vi "NEW Gas Rack MAIN (RT).vi"() -> ()   [LabVIEW 2013]
uses:
  TypeDef/DataCluster.ctl
  TypeDef/Controller Names.ctl
  RT subVIs/Controls/TraceCluster.ctl
  TypeDef/Command Cluster.ctl
  TCP/PC/Event Mode.ctl
  CAN Communication/CAN Mode.ctl
  TCP/RT/RTsend PCrecv CMD.ctl
  RT subVIs/Controls/Stream RT FIFO Mode.ctl
  TypeDef/TCP Cluster.ctl
  TypeDef/Stability Cluster.ctl
  <vilib>/FPGAPlugInAG/sbRIO-9626/niLvFpga_Open_sbRIO-9626.vi
  <vilib>/rvi/interface/common/dynamic/niFpgaDynamicAddResources.vi
  <vilib>/rvi/interface/common/niFpgaWaitOnOcc.vi
  <vilib>/Utility/error.llb/Error Cluster From Error Code.vi
  <vilib>/rvi/errors/niLvFpgaAdjustHostInterfaceError.vi
  <vilib>/FPGAPlugInAG/Dynamic/niLvFpga_Reset_Dynamic.vi
  <vilib>/FPGAPlugInAG/Dynamic/niLvFpga_Run_Dynamic.vi
  <vilib>/rvi/interface/nirviOpenFPGA/nirviOpenFPGA.xnode
  FPGA Bitfiles/New Gas Rack.lvbitx
  FPGA/NEW Gas Rack Main (FPGA).vi
  <vilib>/rvi/interface/nirviReadWriteControl/nirviReadWriteControl.xnode
  <vilib>/rvi/interface/nirviMethod/nirviMethod.xnode
  <vilib>/NI_Real-Time Target Support.lvlib
  <vilib>/rvi/interface/Simulation/niFpgaSimulationCallBeginRW.vi
  <vilib>/ptbypt/NI_PtbyPt.lvlib
  <vilib>/FPGAPlugInAG/Dynamic/niLvFpga_ReadFifo_Dynamic.vi
  <vilib>/rvi/errors/niLvFpgaMergeErrorWithErrorCode.vi
  <vilib>/Analysis/NI_AALBase.lvlib
  <vilib>/Analysis/3filter.llb/Butterworth Filter (DBL).vi
  NiFpgaLv.dll
panel:
  out "element":dbl
  out "output array":dbl[](array[numeric])
  out "x-y":u32
  in  "Load Cmd":bool
  in  "CMD to Load":T1
  out "time 3":dbl
  out "time 2":dbl
  out "time":dbl
  out "Ave Data Cluster":T2 {"Efficiency (%)" format="%#_6f"; "Speed (RPM)" format="%#.1f"; "Fuel Temp (C)" format="%.1f"; "Controller Current (A)" format="%.2f"; "Controller Voltage (V)" format="%.2f"; "Flow (L/H)" format="%.1f"; "Pressure (kPA)" format="%.1f"; "Pump Current (Arms)" format="%.2f"; "Pump Voltage (V)" format="%#.2f"}
  in  "Tab Control Config":enum32{"PID/slew", "Cal/Hidden"}(tab)
  in  "SaveConfig":bool
  in  "ControlArray":T3(array[cluster])
  in  "Cal Coeffs":dbl[][](array[numeric])
  in  "TraceCluster":T4
  out "Speed":dbl
  in  "Max Window":dbl=1400.0 format="%.4f"
  in  "Min Window":dbl=300.0 format="%.4f"
  in  "ave pts":i32=10
  in  "EnumV":enum16{"Pump", "Controller"}(ring)
  in  "CAN CMD":u16
  out "PWM Period (ticks)":u32
  out "Speed Loop Time":dbl
  out "Actual Loop Time 2":u32
  in  "Count 2(uS)":u32=35
  out "Actual Loop Time":u32
  in  "Count 1(uS)":u32=100
  in  "Set Threshold":bool
  in  "Threshold":fxp<+/-,24,7> format="%#_20g"
  in  "Hysteresis":fxp<+,10,6>
  in  "CtCuttoff":fxp<+,24,5>=2.5416698455810547
  in  "Brushed Speed":bool
  in  "Stream Stop":bool
  in  "CommSegs":i32
  out "PrevCalDate":dbl
  in  "CmdCluster":T1
  out "PresSig":dbl
  out "VSig":dbl
  in  "VDirect":dbl
  in  "DirectV?":bool
  in  "DirectPres?":bool
  in  "PresDirect":dbl
  in  "constant update?":bool
  in  "Deadhead?":bool
  in  "PS Enable":bool
  out "Controller Name":T5
  out "Inst Data Cluster":T2 {"Efficiency (%)" format="%.2f"; "Speed (RPM)" format="%#.0f"; "Fuel Temp (C)" format="%.1f"; "Controller Current (A)" format="%.2f"; "Controller Voltage (V)" format="%.2f"; "Flow (L/H)" format="%.1f"; "Pressure (kPA)" format="%.1f"; "Pump Current (Arms)" format="%.2f"; "Pump Voltage (V)" format="%.2f"}
  out "Total (%)":dbl
  in  "GraphTab":enum32{"Page 1", "Page 2"}(tab)
  out "WFG1":dbl[][](graph)
  out "WFG2":dbl[][](graph)
  out "WFG3":dbl[][](graph)
  out "WFG6":dbl[][](graph)
  out "WFG5":dbl[][](graph)
  out "WFG4":dbl[][](graph)
  # "Minimum slew rate is\n600 * step size. This would\nlimit the per cycle change\nto a step size.\n\nChanges were close to expected\nbut changed the PID slews to\nexpected timing rather than\nfinding the time and results\nwere exact.\n\nWas wrong about how the slew\nworks. Slew of 5 still creates\nresults with a stepsize of 0.1.\nIt will just not change every\ncycle but will keep track\nuntil necessary build up."
  # "Should be 0.1"
  # "No longer needed once FPGA is cleaned up"
  # "CalDate is frozen to 3/8/17"
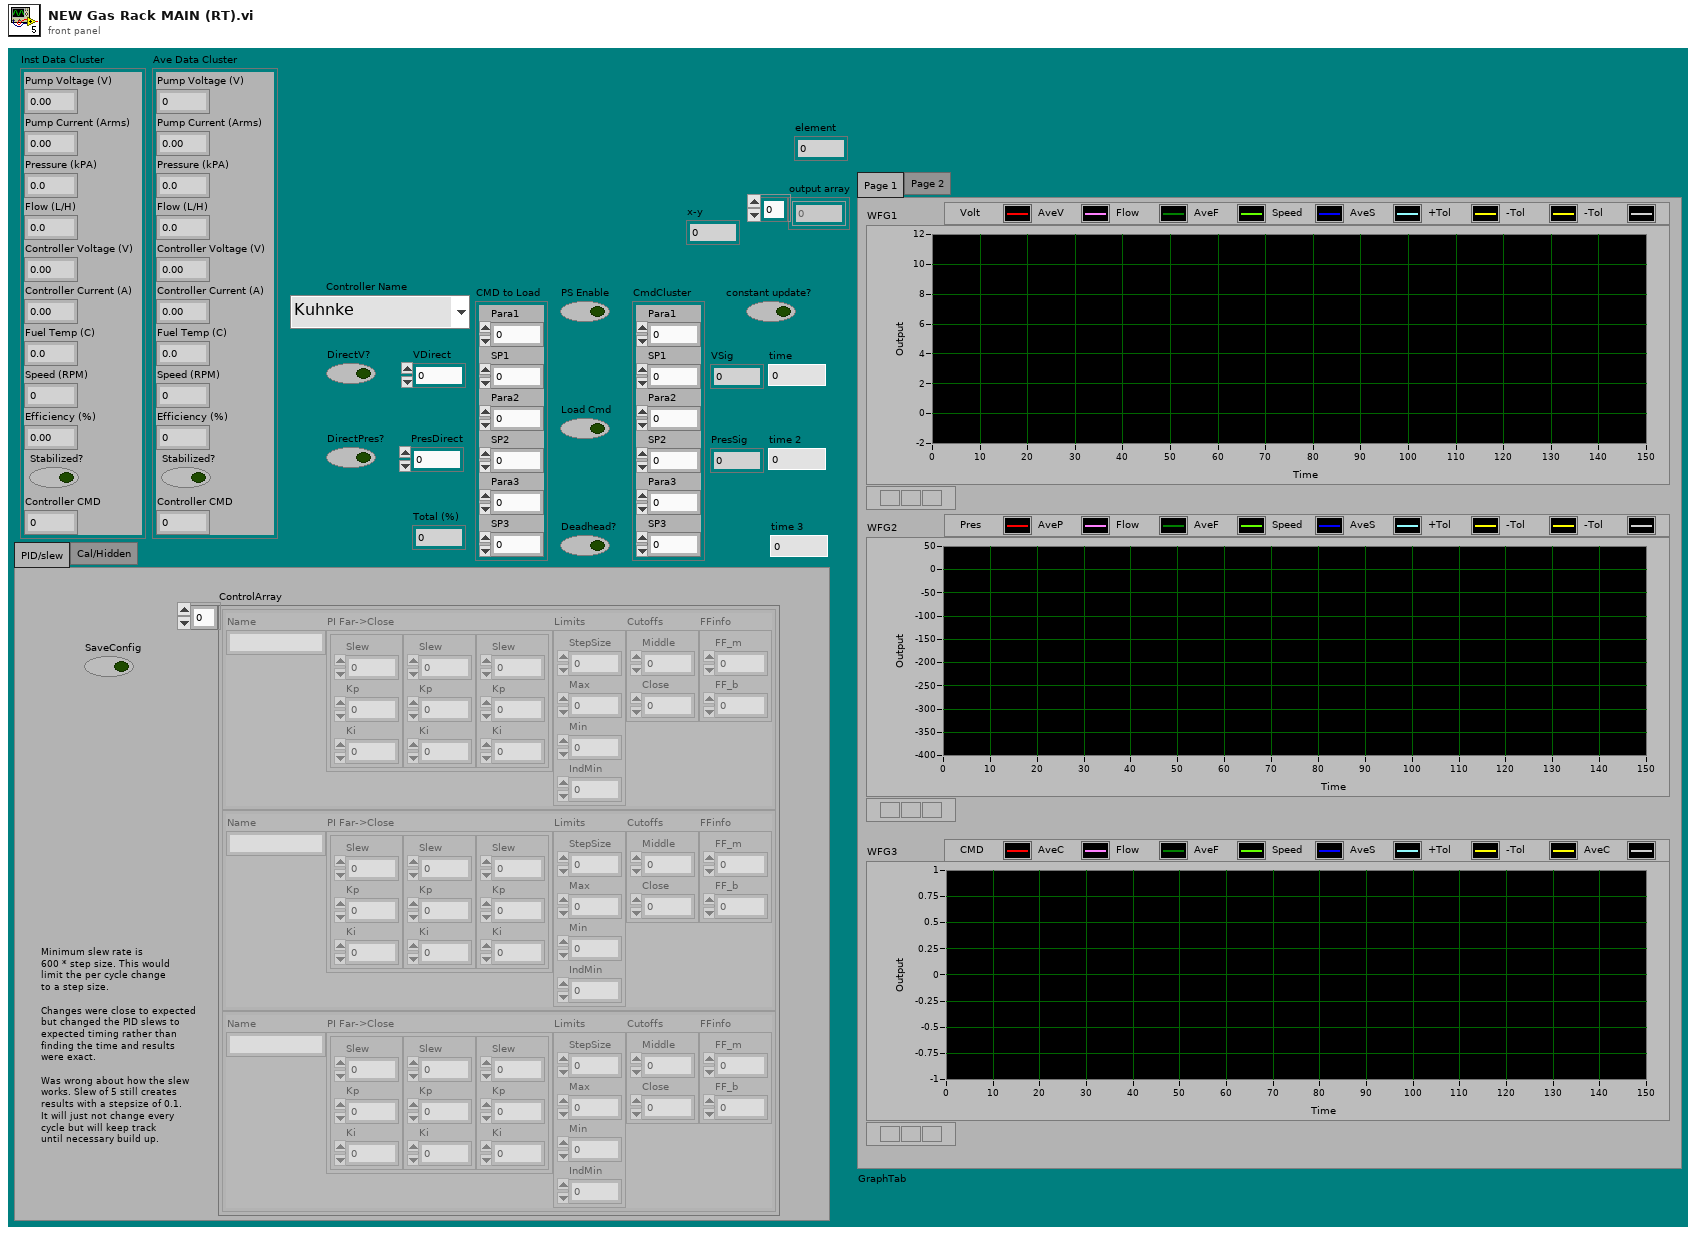
[diagram p1: front panel]
types:
  T1 = typedef "Command Cluster.ctl" = cluster{"Para1":i32, "SP1":dbl, "Para2":i32, "SP2":dbl, "Para3":i32, "SP3":dbl}
  T2 = typedef "DataCluster.ctl" = cluster{"Pump Voltage (V)":dbl, "Pump Current (Arms)":dbl, "Pressure (kPA)":dbl, "Flow (L/H)":dbl, "Controller Voltage (V)":dbl, "Controller Current (A)":dbl, "Fuel Temp (C)":dbl, "Speed (RPM)":dbl, "Efficiency (%)":dbl, "Stabilized?":bool, "Controller CMD":dbl}
  T3 = cluster{"Name":string, "PI Far->Close":cluster{"Slew":dbl, "Kp":dbl, "Ki":dbl}[], "Limits":cluster{"StepSize":dbl, "Max":dbl, "Min":dbl, "IndMin":dbl}, "Cutoffs":cluster{"Middle":dbl, "Close":dbl}, "FFinfo":cluster{"FF_m":dbl, "FF_b":dbl}}[]
  T4 = typedef "TraceCluster.ctl" = cluster{"PreTriggerPts":i32, "TotalPts":i32, "TriggerLvl":dbl, "PlotStyle":enum16{"Single - Rising Edge", "Single - Falling Edge", "Continuous", "Repeat - Rising Edge", "Repeat - Falling Edge"}, "TriggerChannel":i32, "TraceCtrl":bool}
  T5 = typedef "Controller Names.ctl" = enum16{"Kuhnke", "Helbako BLDC", "Conti", "Hella BLDC Screw", "Hella BLDC Turbine", "Helbako (old)", "TI PWM", "PSA", "Hella Gas", "Hella Diesel", "8 Comm", "10 Comm", "8 Comm Hella", "10 Comm Hella", "8 Comm Omron", "10 Comm Omron", "8 Comm Nissan", "10 Comm Nissan"}
  T6 = cluster{"Controller Name":T5, "CommSeg":i32, "PWM?":bool, "Frequency":i32, "Low Command":dbl, "High Command":dbl, "Stop Command":dbl, "Command Step":dbl, "Solenoid Stop?":bool, "Controller?":bool, "Name":string, "Indirect Nonzero CMD":dbl}[]
  T7 = cluster{"Controller Name":T5, "CommSeg":i32, "PWM?":bool, "Frequency":i32, "Low Command":dbl, "High Command":dbl, "Stop Command":dbl, "Command Step":dbl, "Solenoid Stop?":bool, "Controller?":bool, "Name":string, "Indirect Nonzero CMD":dbl}
  T8 = cluster{"Name":string, "PI Far->Close":cluster{"Slew":dbl, "Kp":dbl, "Ki":dbl}[], "Limits":cluster{"StepSize":dbl, "Max":dbl, "Min":dbl}, "Cutoffs":cluster{"Middle":dbl, "Close":dbl}, "FFinfo":cluster{"FF_m":dbl, "FF_b":dbl}}[]
  T9 = cluster{"Stability Reads":i32, "Stability1":i32, "Stability2":i32, "Stability3":i32}
  T10 = typedef "RTsend PCrecv CMD.ctl" = enum16{"Data", "Connected?", "CalFileDate"}
  T11 = typedef "CAN Mode.ctl" = enum16{"Init", "Read", "Write", "Close"}
  T12 = typedef "Event Mode.ctl" = enum16{"Init", "Get", "Set", "Destroy"}
  T13 = cluster{"CommandCluster":T1, "Deadhead?":bool, "PI Rate (sec)":dbl, "PI Timer":dbl, "FPGA Data Rate (sec)":dbl, "FPGA Data Timer":dbl, "PC Data Rate (sec)":dbl, "PC Data Timer":dbl, "InstDataCluster":T2, "Controller":cluster{"Controller Name":T5, "CommSeg":i32, "PWM?":bool, "Frequency":i32, "Low Command":dbl, "High Command":dbl, "Stop Command":dbl, "Command Step":dbl, "Solenoid Stop?":bool, "Controller?":bool, "Name":string, "Indirect Nonzero CMD":dbl}, "PWM Period (ticks)":u32, "Tolerances":dbl[], "Cal Coeffs":dbl[][], "EnumV":enum16{"Pump", "Controller"}, "PS Enable":bool, "StabilityCluster":cluster{"Stability Reads":i32, "Stability1":i32, "Stability2":i32, "Stability3":i32}, "AveDataCluster":T2, "CMD Scaler":dbl, "ControlArray":cluster{"Name":string, "PI Far->Close":cluster{"Slew":dbl, "Kp":dbl, "Ki":dbl}[], "Limits":cluster{"StepSize":dbl, "Max":dbl, "Min":dbl, "IndMin":dbl}, "Cutoffs":cluster{"Middle":dbl, "Close":dbl}, "FFinfo":cluster{"FF_m":dbl, "FF_b":dbl}}[], "Controller List":cluster{"Controller Name":T5, "CommSeg":i32, "PWM?":bool, "Frequency":i32, "Low Command":dbl, "High Command":dbl, "Stop Command":dbl, "Command Step":dbl, "Solenoid Stop?":bool, "Controller?":bool, "Name":string, "Indirect Nonzero CMD":dbl}[], "VandPLimit":dbl[]}
  T14 = typedef "TCP Cluster.ctl" = cluster{"Command":string, "FlattenedData":string}
  T15 = typedef "Stream RT FIFO Mode.ctl" = enum16{"Create", "Write", "Read", "Delete"}
  T16 = typedef "PCsend RTrecv CMD.ctl" = enum16{"ConnSettings", "Connect", "CMD", "Controller", "PSenable", "ReqCalDate", "Tolerances", "Stable Trigger", "Stop", "VPLimits"}
  T17 = typedef "Stability Cluster.ctl" = cluster{"Voltage Tolerances":dbl, "Pressure Tolerances":dbl, "Flow Tolerances":dbl, "Speed Tolerances":dbl, "Stable Count (sec)":dbl}
  T18 = cluster{"Pump Voltage":fxp<+/-,25,15>, "Pump Current":fxp<+/-,25,15>, "Pressure":fxp<+/-,25,15>, "Flow":fxp<+/-,25,15>, "Controller Voltage":fxp<+/-,25,15>, "Controller Current":fxp<+/-,25,15>, "Temperature":fxp<+/-,25,15>, "Speed":fxp<+/-,25,15>}
  T19 = cluster{"[0]":dbl, "[1]":dbl, "[2]":dbl, "[3]":dbl, "[4]":dbl, "[5]":dbl, "[6]":dbl, "[7]":dbl}
  T20 = typedef "NI_Real-Time Target Support.lvlib/RT CPU Load.ctl" = cluster{"Total (%)":dbl, "Time Critical (%)":dbl, "Timed Structures (%)":dbl, "High (%)":dbl, "Above Normal (%)":dbl, "Normal (%)":dbl, "Background (%)":dbl, "Idle (%)":dbl, "ISR (%)":dbl}
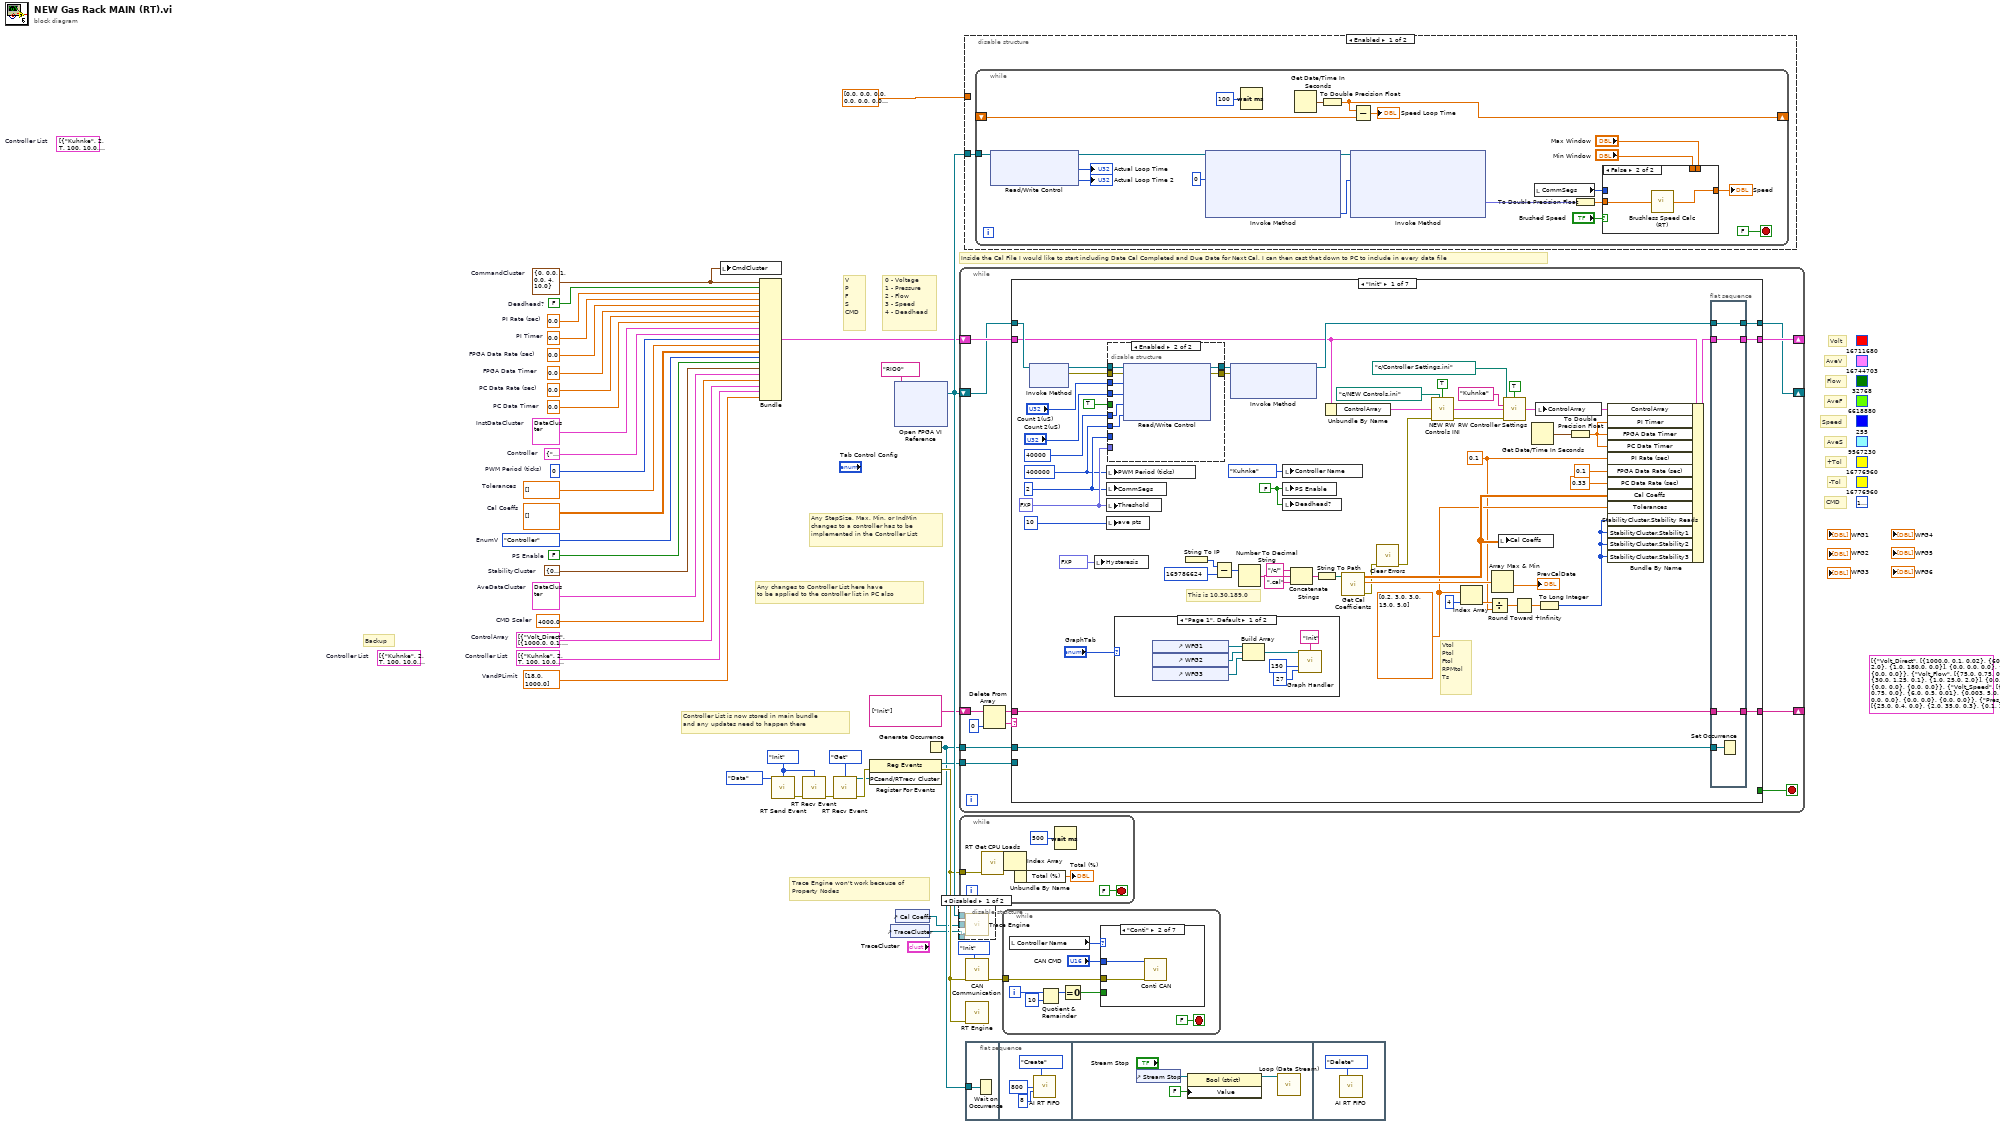
[diagram p0: block diagram]
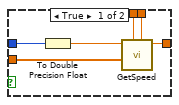
[diagram p2: hidden frame]
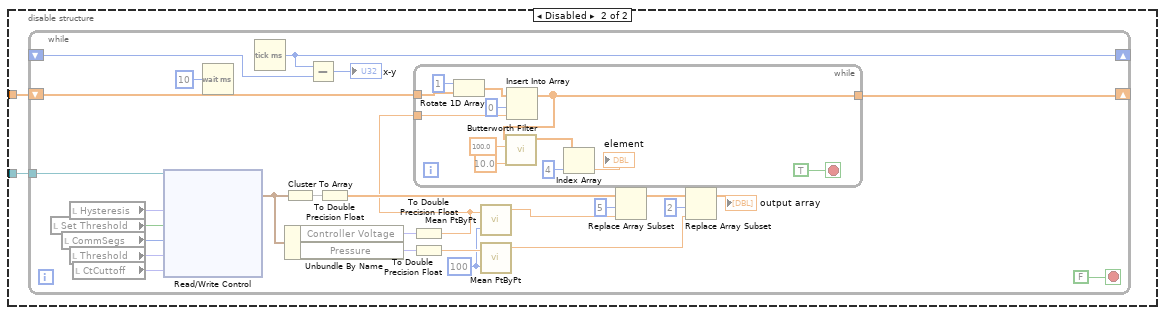
[diagram p3: hidden frame]
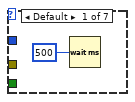
[diagram p5: hidden frame]
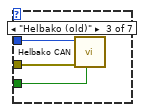
[diagram p6: hidden frame]
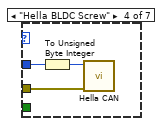
[diagram p7: hidden frame]
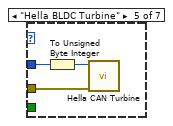
[diagram p8: hidden frame]
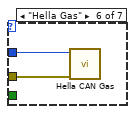
[diagram p9: hidden frame]
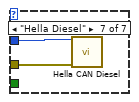
[diagram p10: hidden frame]
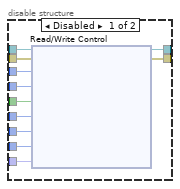
[diagram p11: hidden frame]
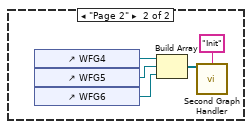
[diagram p12: hidden frame]
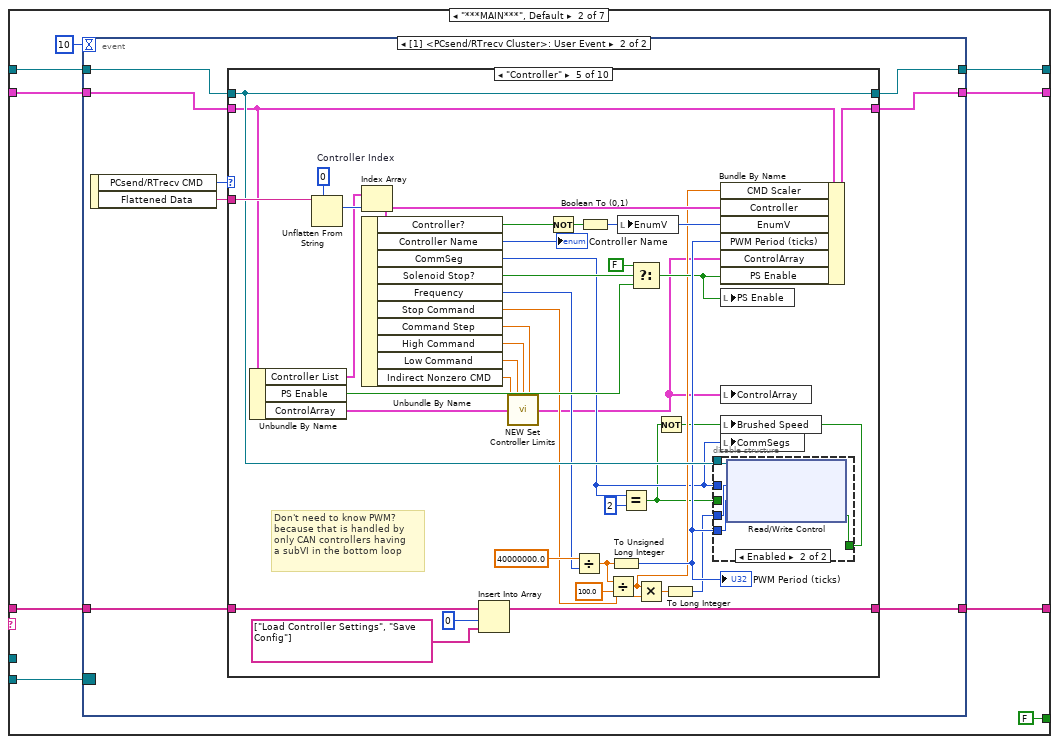
[diagram p13: hidden frame]
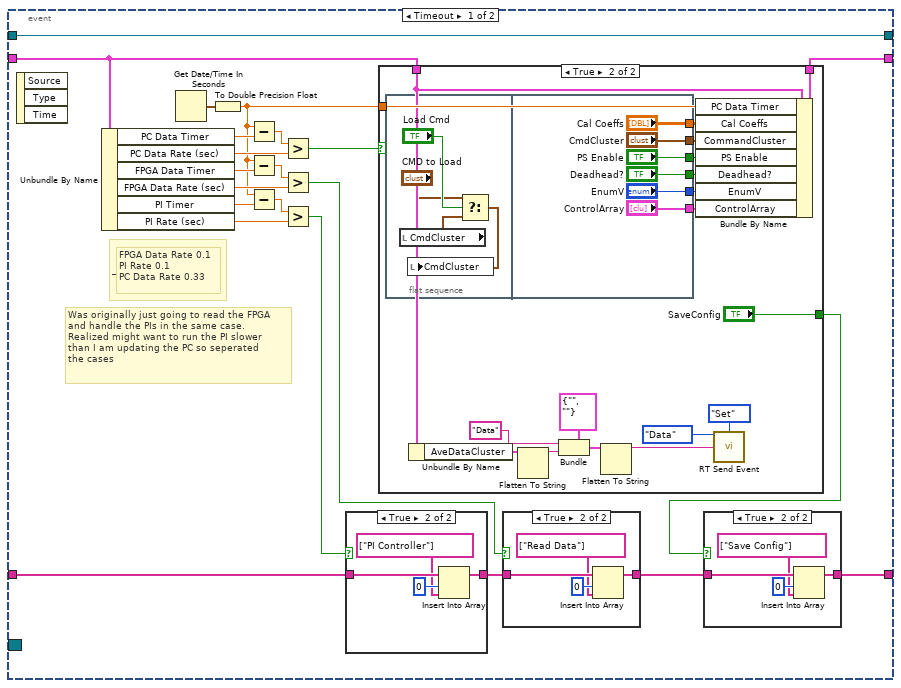
[diagram p14: hidden frame]
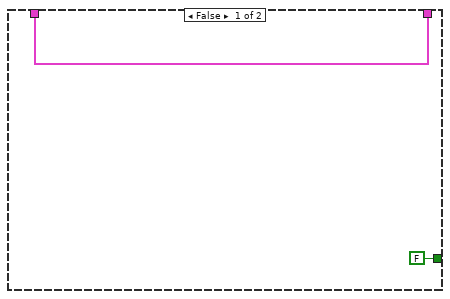
[diagram p18: hidden frame]
diagram:
  (unwired) T6 [{"Controller Name"=enum."Kuhnke", "CommSeg"=2, "PWM?"=TRUE, "Frequency"=100, "Low Command"=10.0, "High Command"=90.0, "Stop Command"=10.0, "Command Step"=0.1, "Solenoid Stop?"=FALSE, "Controller?"=TRUE, "Name"="Kuhnke", "Indirect Nonzero CMD"=15.0}, {"Controller Name"=enum."Helbako BLDC", "CommSeg"=2, "PWM?"=TRUE, "Frequency"=100, "Low Command"=10.0, "High Command"=90.0, "Stop Command"=10.0, "Command Step"=0.1, "Solenoid Stop?"=FALSE, "Controller?"=TRUE, "Name"="Helbako BLDC", "Indirect Nonzero CMD"=15.0}, {"Controller Name"=enum."Conti", "CommSeg"=2, "PWM?"=FALSE, "Frequency"=100, "Low Command"=0.0, "High Command"=800.0, "Stop Command"=0.0, "Command Step"=1.0, "Solenoid Stop?"=FALSE, "Controller?"=TRUE, "Name"="Conti", "Indirect Nonzero CMD"=0.0}, {"Controller Name"=enum."Hella BLDC Screw", "CommSeg"=2, "PWM?"=FALSE, "Frequency"=100, "Low Command"=0.0, "High Command"=100.0, "Stop Command"=0.0, "Command Step"=1.0, "Solenoid Stop?"=FALSE, "Controller?"=TRUE, "Name"="Hella BLDC Screw", "Indirect Nonzero CMD"=10.0}, {"Controller Name"=enum."Hella BLDC Turbine", "CommSeg"=2, "PWM?"=FALSE, "Frequency"=100, "Low Command"=0.0, "High Command"=100.0, "Stop Command"=0.0, "Command Step"=1.0, "Solenoid Stop?"=FALSE, "Controller?"=TRUE, "Name"="Hella BLDC Turbine", "Indirect Nonzero CMD"=10.0}, {"Controller Name"=enum."Helbako (old)", "CommSeg"=2, "PWM?"=FALSE, "Frequency"=100, "Low Command"=0.0, "High Command"=100.0, "Stop Command"=0.0, "Command Step"=0.1, "Solenoid Stop?"=FALSE, "Controller?"=TRUE, "Name"="Helbako (old)", "Indirect Nonzero CMD"=0.0}, {"Controller Name"=enum."TI PWM", "CommSeg"=2, "PWM?"=TRUE, "Frequency"=100, "Low Command"=0.0, "High Command"=100.0, "Stop Command"=0.0, "Command Step"=0.1, "Solenoid Stop?"=FALSE, "Controller?"=TRUE, "Name"="TI PWM", "Indirect Nonzero CMD"=0.0}, {"Controller Name"=enum."PSA", "CommSeg"=2, "PWM?"=TRUE, "Frequency"=100, "Low Command"=5.0, "High Command"=95.0, "Stop Command"=5.0, "Command Step"=0.1, "Solenoid Stop?"=FALSE, "Controller?"=TRUE, "Name"="PSA", "Indirect Nonzero CMD"=5.0}, {"Controller Name"=enum."Hella Gas", "CommSeg"=2, "PWM?"=FALSE, "Frequency"=100, "Low Command"=0.0, "High Command"=800.0, "Stop Command"=0.0, "Command Step"=1.0, "Solenoid Stop?"=TRUE, "Controller?"=TRUE, "Name"="Hella Gas", "Indirect Nonzero CMD"=0.0}, {"Controller Name"=enum."Hella Diesel", "CommSeg"=10, "PWM?"=FALSE, "Frequency"=100, "Low Command"=370.0, "High Command"=461.0, "Stop Command"=370.0, "Command Step"=1.0, "Solenoid Stop?"=TRUE, "Controller?"=TRUE, "Name"="Hella Diesel", "Indirect Nonzero CMD"=370.0}, {"Controller Name"=enum."8 Comm", "CommSeg"=8, "PWM?"=FALSE, "Frequency"=150, "Low Command"=0.0, "High Command"=1.0, "Stop Command"=0.0, "Command Step"=1.0, "Solenoid Stop?"=FALSE, "Controller?"=FALSE, "Name"="8 Comm", "Indirect Nonzero CMD"=0.0}, {"Controller Name"=enum."10 Comm", "CommSeg"=10, "PWM?"=FALSE, "Frequency"=150, "Low Command"=0.0, "High Command"=1.0, "Stop Command"=0.0, "Command Step"=1.0, "Solenoid Stop?"=FALSE, "Controller?"=FALSE, "Name"="10 Comm", "Indirect Nonzero CMD"=0.0}, {"Controller Name"=enum."8 Comm Hella", "CommSeg"=8, "PWM?"=TRUE, "Frequency"=150, "Low Command"=0.0, "High Command"=50.0, "Stop Command"=80.0, "Command Step"=0.1, "Solenoid Stop?"=FALSE, "Controller?"=TRUE, "Name"="8 Comm Hella", "Indirect Nonzero CMD"=0.0}, {"Controller Name"=enum."10 Comm Hella", "CommSeg"=10, "PWM?"=TRUE, "Frequency"=150, "Low Command"=0.0, "High Command"=50.0, "Stop Command"=80.0, "Command Step"=0.1, "Solenoid Stop?"=FALSE, "Controller?"=TRUE, "Name"="10 Comm Hella", "Indirect Nonzero CMD"=0.0}, {"Controller Name"=enum."8 Comm Omron", "CommSeg"=8, "PWM?"=TRUE, "Frequency"=150, "Low Command"=5.0, "High Command"=50.0, "Stop Command"=75.0, "Command Step"=0.1, "Solenoid Stop?"=FALSE, "Controller?"=TRUE, "Name"="8 Comm Omron", "Indirect Nonzero CMD"=5.0}, {"Controller Name"=enum."10 Comm Omron", "CommSeg"=10, "PWM?"=TRUE, "Frequency"=150, "Low Command"=5.0, "High Command"=50.0, "Stop Command"=75.0, "Command Step"=0.1, "Solenoid Stop?"=FALSE, "Controller?"=TRUE, "Name"="10 Comm Omron", "Indirect Nonzero CMD"=5.0}, {"Controller Name"=enum."8 Comm Nissan", "CommSeg"=8, "PWM?"=TRUE, "Frequency"=10, "Low Command"=50.0, "High Command"=90.0, "Stop Command"=50.0, "Command Step"=0.1, "Solenoid Stop?"=TRUE, "Controller?"=TRUE, "Name"="8 Comm Nissan", "Indirect Nonzero CMD"=50.0}, {"Controller Name"=enum."10 Comm Nissan", "CommSeg"=10, "PWM?"=TRUE, "Frequency"=10, "Low Command"=50.0, "High Command"=90.0, "Stop Command"=50.0, "Command Step"=0.1, "Solenoid Stop?"=TRUE, "Controller?"=TRUE, "Name"="10 Comm Nissan", "Indirect Nonzero CMD"=50.0}]  # Controller List
  w2 = T6 [{"Controller Name"=enum."Kuhnke", "CommSeg"=2, "PWM?"=TRUE, "Frequency"=100, "Low Command"=10.0, "High Command"=90.0, "Stop Command"=10.0, "Command Step"=0.1, "Solenoid Stop?"=FALSE, "Controller?"=TRUE, "Name"="Kuhnke", "Indirect Nonzero CMD"=15.0}, {"Controller Name"=enum."Helbako BLDC", "CommSeg"=2, "PWM?"=TRUE, "Frequency"=100, "Low Command"=10.0, "High Command"=90.0, "Stop Command"=10.0, "Command Step"=0.1, "Solenoid Stop?"=FALSE, "Controller?"=TRUE, "Name"="Helbako BLDC", "Indirect Nonzero CMD"=15.0}, {"Controller Name"=enum."Conti", "CommSeg"=2, "PWM?"=FALSE, "Frequency"=100, "Low Command"=0.0, "High Command"=800.0, "Stop Command"=0.0, "Command Step"=1.0, "Solenoid Stop?"=FALSE, "Controller?"=TRUE, "Name"="Conti", "Indirect Nonzero CMD"=0.0}, {"Controller Name"=enum."Hella BLDC Screw", "CommSeg"=2, "PWM?"=FALSE, "Frequency"=100, "Low Command"=0.0, "High Command"=100.0, "Stop Command"=0.0, "Command Step"=1.0, "Solenoid Stop?"=FALSE, "Controller?"=TRUE, "Name"="Hella BLDC Screw", "Indirect Nonzero CMD"=10.0}, {"Controller Name"=enum."Hella BLDC Turbine", "CommSeg"=2, "PWM?"=FALSE, "Frequency"=100, "Low Command"=0.0, "High Command"=100.0, "Stop Command"=0.0, "Command Step"=1.0, "Solenoid Stop?"=FALSE, "Controller?"=TRUE, "Name"="Hella BLDC Turbine", "Indirect Nonzero CMD"=10.0}, {"Controller Name"=enum."Helbako (old)", "CommSeg"=2, "PWM?"=FALSE, "Frequency"=100, "Low Command"=0.0, "High Command"=100.0, "Stop Command"=0.0, "Command Step"=0.1, "Solenoid Stop?"=FALSE, "Controller?"=TRUE, "Name"="Helbako (old)", "Indirect Nonzero CMD"=0.0}, {"Controller Name"=enum."TI PWM", "CommSeg"=2, "PWM?"=TRUE, "Frequency"=100, "Low Command"=0.0, "High Command"=100.0, "Stop Command"=0.0, "Command Step"=0.1, "Solenoid Stop?"=FALSE, "Controller?"=TRUE, "Name"="TI PWM", "Indirect Nonzero CMD"=0.0}, {"Controller Name"=enum."PSA", "CommSeg"=2, "PWM?"=TRUE, "Frequency"=100, "Low Command"=5.0, "High Command"=95.0, "Stop Command"=5.0, "Command Step"=0.1, "Solenoid Stop?"=FALSE, "Controller?"=TRUE, "Name"="PSA", "Indirect Nonzero CMD"=5.0}, {"Controller Name"=enum."Hella Gas", "CommSeg"=2, "PWM?"=FALSE, "Frequency"=100, "Low Command"=0.0, "High Command"=800.0, "Stop Command"=0.0, "Command Step"=1.0, "Solenoid Stop?"=TRUE, "Controller?"=TRUE, "Name"="Hella Gas", "Indirect Nonzero CMD"=0.0}, {"Controller Name"=enum."Hella Diesel", "CommSeg"=10, "PWM?"=FALSE, "Frequency"=100, "Low Command"=370.0, "High Command"=461.0, "Stop Command"=370.0, "Command Step"=1.0, "Solenoid Stop?"=TRUE, "Controller?"=TRUE, "Name"="Hella Diesel", "Indirect Nonzero CMD"=370.0}, {"Controller Name"=enum."8 Comm", "CommSeg"=8, "PWM?"=FALSE, "Frequency"=150, "Low Command"=0.0, "High Command"=1.0, "Stop Command"=0.0, "Command Step"=1.0, "Solenoid Stop?"=FALSE, "Controller?"=FALSE, "Name"="8 Comm", "Indirect Nonzero CMD"=0.0}, {"Controller Name"=enum."10 Comm", "CommSeg"=10, "PWM?"=FALSE, "Frequency"=150, "Low Command"=0.0, "High Command"=1.0, "Stop Command"=0.0, "Command Step"=1.0, "Solenoid Stop?"=FALSE, "Controller?"=FALSE, "Name"="10 Comm", "Indirect Nonzero CMD"=0.0}, {"Controller Name"=enum."8 Comm Hella", "CommSeg"=8, "PWM?"=TRUE, "Frequency"=150, "Low Command"=0.0, "High Command"=50.0, "Stop Command"=80.0, "Command Step"=0.1, "Solenoid Stop?"=FALSE, "Controller?"=TRUE, "Name"="8 Comm Hella", "Indirect Nonzero CMD"=0.0}, {"Controller Name"=enum."10 Comm Hella", "CommSeg"=10, "PWM?"=TRUE, "Frequency"=150, "Low Command"=0.0, "High Command"=50.0, "Stop Command"=80.0, "Command Step"=0.1, "Solenoid Stop?"=FALSE, "Controller?"=TRUE, "Name"="10 Comm Hella", "Indirect Nonzero CMD"=0.0}, {"Controller Name"=enum."8 Comm Omron", "CommSeg"=8, "PWM?"=TRUE, "Frequency"=150, "Low Command"=5.0, "High Command"=50.0, "Stop Command"=75.0, "Command Step"=0.1, "Solenoid Stop?"=FALSE, "Controller?"=TRUE, "Name"="8 Comm Omron", "Indirect Nonzero CMD"=5.0}, {"Controller Name"=enum."10 Comm Omron", "CommSeg"=10, "PWM?"=TRUE, "Frequency"=150, "Low Command"=5.0, "High Command"=50.0, "Stop Command"=75.0, "Command Step"=0.1, "Solenoid Stop?"=FALSE, "Controller?"=TRUE, "Name"="10 Comm Omron", "Indirect Nonzero CMD"=5.0}, {"Controller Name"=enum."8 Comm Nissan", "CommSeg"=8, "PWM?"=TRUE, "Frequency"=10, "Low Command"=50.0, "High Command"=90.0, "Stop Command"=50.0, "Command Step"=0.1, "Solenoid Stop?"=TRUE, "Controller?"=TRUE, "Name"="8 Comm Nissan", "Indirect Nonzero CMD"=50.0}, {"Controller Name"=enum."10 Comm Nissan", "CommSeg"=10, "PWM?"=TRUE, "Frequency"=10, "Low Command"=50.0, "High Command"=90.0, "Stop Command"=50.0, "Command Step"=0.1, "Solenoid Stop?"=TRUE, "Controller?"=TRUE, "Name"="10 Comm Nissan", "Indirect Nonzero CMD"=50.0}]  # Controller List
  (unwired) T6 [{"Controller Name"=enum."Kuhnke", "CommSeg"=2, "PWM?"=TRUE, "Frequency"=100, "Low Command"=10.0, "High Command"=90.0, "Stop Command"=10.0, "Command Step"=0.1, "Solenoid Stop?"=FALSE, "Controller?"=TRUE, "Name"="Kuhnke", "Indirect Nonzero CMD"=15.0}, {"Controller Name"=enum."Helbako BLDC", "CommSeg"=2, "PWM?"=TRUE, "Frequency"=100, "Low Command"=10.0, "High Command"=90.0, "Stop Command"=10.0, "Command Step"=0.1, "Solenoid Stop?"=FALSE, "Controller?"=TRUE, "Name"="Helbako BLDC", "Indirect Nonzero CMD"=15.0}, {"Controller Name"=enum."Conti", "CommSeg"=2, "PWM?"=FALSE, "Frequency"=100, "Low Command"=0.0, "High Command"=800.0, "Stop Command"=0.0, "Command Step"=1.0, "Solenoid Stop?"=FALSE, "Controller?"=TRUE, "Name"="Conti", "Indirect Nonzero CMD"=0.0}, {"Controller Name"=enum."Hella BLDC Screw", "CommSeg"=2, "PWM?"=FALSE, "Frequency"=100, "Low Command"=0.0, "High Command"=100.0, "Stop Command"=0.0, "Command Step"=0.1, "Solenoid Stop?"=FALSE, "Controller?"=TRUE, "Name"="Hella BLDC", "Indirect Nonzero CMD"=0.0}, {"Controller Name"=enum."Helbako (old)", "CommSeg"=2, "PWM?"=FALSE, "Frequency"=100, "Low Command"=0.0, "High Command"=100.0, "Stop Command"=0.0, "Command Step"=0.1, "Solenoid Stop?"=FALSE, "Controller?"=TRUE, "Name"="Helbako (old)", "Indirect Nonzero CMD"=0.0}, {"Controller Name"=enum."TI PWM", "CommSeg"=2, "PWM?"=TRUE, "Frequency"=100, "Low Command"=0.0, "High Command"=100.0, "Stop Command"=0.0, "Command Step"=0.1, "Solenoid Stop?"=FALSE, "Controller?"=TRUE, "Name"="TI PWM", "Indirect Nonzero CMD"=0.0}, {"Controller Name"=enum."PSA", "CommSeg"=2, "PWM?"=TRUE, "Frequency"=100, "Low Command"=5.0, "High Command"=95.0, "Stop Command"=5.0, "Command Step"=0.1, "Solenoid Stop?"=FALSE, "Controller?"=TRUE, "Name"="PSA", "Indirect Nonzero CMD"=5.0}, {"Controller Name"=enum."Hella Gas", "CommSeg"=2, "PWM?"=FALSE, "Frequency"=100, "Low Command"=0.0, "High Command"=800.0, "Stop Command"=0.0, "Command Step"=1.0, "Solenoid Stop?"=TRUE, "Controller?"=TRUE, "Name"="Hella Gas", "Indirect Nonzero CMD"=0.0}, {"Controller Name"=enum."Hella Diesel", "CommSeg"=10, "PWM?"=FALSE, "Frequency"=100, "Low Command"=370.0, "High Command"=461.0, "Stop Command"=370.0, "Command Step"=1.0, "Solenoid Stop?"=TRUE, "Controller?"=TRUE, "Name"="Hella Diesel", "Indirect Nonzero CMD"=370.0}, {"Controller Name"=enum."8 Comm", "CommSeg"=8, "PWM?"=FALSE, "Frequency"=150, "Low Command"=0.0, "High Command"=1.0, "Stop Command"=0.0, "Command Step"=1.0, "Solenoid Stop?"=FALSE, "Controller?"=FALSE, "Name"="8 Comm", "Indirect Nonzero CMD"=0.0}, {"Controller Name"=enum."10 Comm", "CommSeg"=10, "PWM?"=FALSE, "Frequency"=150, "Low Command"=0.0, "High Command"=1.0, "Stop Command"=0.0, "Command Step"=1.0, "Solenoid Stop?"=FALSE, "Controller?"=FALSE, "Name"="10 Comm", "Indirect Nonzero CMD"=0.0}, {"Controller Name"=enum."8 Comm Hella", "CommSeg"=8, "PWM?"=TRUE, "Frequency"=150, "Low Command"=0.0, "High Command"=50.0, "Stop Command"=80.0, "Command Step"=0.1, "Solenoid Stop?"=FALSE, "Controller?"=TRUE, "Name"="8 Comm Hella", "Indirect Nonzero CMD"=0.0}, {"Controller Name"=enum."10 Comm Hella", "CommSeg"=10, "PWM?"=TRUE, "Frequency"=150, "Low Command"=0.0, "High Command"=50.0, "Stop Command"=80.0, "Command Step"=0.1, "Solenoid Stop?"=FALSE, "Controller?"=TRUE, "Name"="10 Comm Hella", "Indirect Nonzero CMD"=0.0}, {"Controller Name"=enum."8 Comm Omron", "CommSeg"=8, "PWM?"=TRUE, "Frequency"=150, "Low Command"=5.0, "High Command"=50.0, "Stop Command"=75.0, "Command Step"=0.1, "Solenoid Stop?"=FALSE, "Controller?"=TRUE, "Name"="8 Comm Omron", "Indirect Nonzero CMD"=5.0}, {"Controller Name"=enum."10 Comm Omron", "CommSeg"=10, "PWM?"=TRUE, "Frequency"=150, "Low Command"=5.0, "High Command"=50.0, "Stop Command"=75.0, "Command Step"=0.1, "Solenoid Stop?"=FALSE, "Controller?"=TRUE, "Name"="10 Comm Omron", "Indirect Nonzero CMD"=5.0}, {"Controller Name"=enum."8 Comm Nissan", "CommSeg"=8, "PWM?"=TRUE, "Frequency"=10, "Low Command"=50.0, "High Command"=90.0, "Stop Command"=50.0, "Command Step"=0.1, "Solenoid Stop?"=TRUE, "Controller?"=TRUE, "Name"="8 Comm Nissan", "Indirect Nonzero CMD"=50.0}, {"Controller Name"=enum."10 Comm Nissan", "CommSeg"=10, "PWM?"=TRUE, "Frequency"=10, "Low Command"=50.0, "High Command"=90.0, "Stop Command"=50.0, "Command Step"=0.1, "Solenoid Stop?"=TRUE, "Controller?"=TRUE, "Name"="10 Comm Nissan", "Indirect Nonzero CMD"=50.0}]  # Controller List
  w3 = T3 [{"Name"="Volt_Direct", "PI Far->Close"=[{"Slew"=1000.0, "Kp"=0.1, "Ki"=0.02}, {"Slew"=60.0, "Kp"=5.0, "Ki"=2.0}, {"Slew"=1.0, "Kp"=180.0, "Ki"=0.0}], "Limits"={"StepSize"=1e-05, "Max"=10.0, "Min"=0.0, "IndMin"=0.0}, "Cutoffs"={"Middle"=1.5, "Close"=0.2}, "FFinfo"={"FF_m"=0.5, "FF_b"=0.0}}, {"Name"="Volt_Flow", "PI Far->Close"=[{"Slew"=75.0, "Kp"=0.75, "Ki"=0.0}, {"Slew"=30.0, "Kp"=1.25, "Ki"=0.1}, {"Slew"=1.0, "Kp"=25.0, "Ki"=2.0}], "Limits"={"StepSize"=1e-05, "Max"=10.0, "Min"=0.0, "IndMin"=0.0}, "Cutoffs"={"Middle"=15.0, "Close"=4.0}, "FFinfo"={"FF_m"=0.0, "FF_b"=0.0}}, {"Name"="Volt_Speed", "PI Far->Close"=[{"Slew"=200.0, "Kp"=0.75, "Ki"=0.0}, {"Slew"=6.0, "Kp"=0.5, "Ki"=0.01}, {"Slew"=0.003, "Kp"=5.0, "Ki"=3.0}], "Limits"={"StepSize"=1e-05, "Max"=10.0, "Min"=0.0, "IndMin"=0.0}, "Cutoffs"={"Middle"=250.0, "Close"=25.0}, "FFinfo"={"FF_m"=0.0014, "FF_b"=8.5}}, {"Name"="Pres_Direct", "PI Far->Close"=[{"Slew"=25.0, "Kp"=0.4, "Ki"=0.0}, {"Slew"=2.0, "Kp"=35.0, "Ki"=0.3}, {"Slew"=0.1, "Kp"=35.0, "Ki"=0.3}], "Limits"={"StepSize"=1e-05, "Max"=5.0, "Min"=0.0, "IndMin"=0.0}, "Cutoffs"={"Middle"=30.0, "Close"=4.0}, "FFinfo"={"FF_m"=0.0, "FF_b"=0.0}}, {"Name"="Pres_Flow", "PI Far->Close"=[{"Slew"=65.0, "Kp"=-5.0, "Ki"=-10.0}, {"Slew"=25.0, "Kp"=-25.0, "Ki"=-1.0}, {"Slew"=1.0, "Kp"=-250.0, "Ki"=-120.0}], "Limits"={"StepSize"=1e-05, "Max"=5.0, "Min"=0.0, "IndMin"=0.0}, "Cutoffs"={"Middle"=15.0, "Close"=4.0}, "FFinfo"={"FF_m"=0.0, "FF_b"=0.0}}, {"Name"="Pres_Speed", "PI Far->Close"=[{"Slew"=50.0, "Kp"=-100.0, "Ki"=-10.0}, {"Slew"=1.0, "Kp"=-50.0, "Ki"=-7.5}, {"Slew"=1.0, "Kp"=-50.0, "Ki"=-7.5}], "Limits"={"StepSize"=1e-05, "Max"=5.0, "Min"=0.0, "IndMin"=0.0}, "Cutoffs"={"Middle"=250.0, "Close"=25.0}, "FFinfo"={"FF_m"=0.0, "FF_b"=0.0}}, {"Name"="CMD_Direct", "PI Far->Close"=[{"Slew"=1.0, "Kp"=1.0, "Ki"=0.1}, {"Slew"=1.0, "Kp"=1.0, "Ki"=0.1}, {"Slew"=1.0, "Kp"=1.0, "Ki"=0.1}], "Limits"={"StepSize"=0.1, "Max"=90.0, "Min"=10.0, "IndMin"=10.0}, "Cutoffs"={"Middle"=0.0, "Close"=0.0}, "FFinfo"={"FF_m"=1.0, "FF_b"=0.0}}, {"Name"="CMD_Flow", "PI Far->Close"=[{"Slew"=650.0, "Kp"=10.0, "Ki"=1.0}, {"Slew"=50.0, "Kp"=100.0, "Ki"=2.0}, {"Slew"=10.0, "Kp"=140.0, "Ki"=5.0}], "Limits"={"StepSize"=0.1, "Max"=90.0, "Min"=10.0, "IndMin"=15.0}, "Cutoffs"={"Middle"=15.0, "Close"=4.0}, "FFinfo"={"FF_m"=0.0, "FF_b"=90.0}}, {"Name"="CMD_Speed", "PI Far->Close"=[{"Slew"=999999.0, "Kp"=0.0, "Ki"=0.0}, {"Slew"=999999.0, "Kp"=0.0, "Ki"=0.0}, {"Slew"=999999.0, "Kp"=0.15, "Ki"=0.0}], "Limits"={"StepSize"=0.1, "Max"=90.0, "Min"=10.0, "IndMin"=15.0}, "Cutoffs"={"Middle"=250.0, "Close"=25.0}, "FFinfo"={"FF_m"=0.00875, "FF_b"=-2.5}}]  # ControlArray
  w4 = T7 {"Controller Name"=enum."Kuhnke", "CommSeg"=2, "PWM?"=TRUE, "Frequency"=100, "Low Command"=10.0, "High Command"=100.0, "Stop Command"=10.0, "Command Step"=0.1, "Solenoid Stop?"=FALSE, "Controller?"=TRUE, "Name"="Kuhnke", "Indirect Nonzero CMD"=15.0}  # Controller
  w5 = dbl[] [18.0, 1000.0]  # VandPLimit
  (unwired) T8 [{"Name"="Volt_Direct", "PI Far->Close"=[{"Slew"=1000.0, "Kp"=0.1, "Ki"=0.02}, {"Slew"=60.0, "Kp"=5.0, "Ki"=2.0}, {"Slew"=1.0, "Kp"=180.0, "Ki"=0.0}], "Limits"={"StepSize"=0.0, "Max"=0.0, "Min"=0.0}, "Cutoffs"={"Middle"=0.0, "Close"=0.0}, "FFinfo"={"FF_m"=0.0, "FF_b"=0.0}}, {"Name"="Volt_Flow", "PI Far->Close"=[{"Slew"=75.0, "Kp"=0.75, "Ki"=0.0}, {"Slew"=30.0, "Kp"=1.25, "Ki"=0.1}, {"Slew"=1.0, "Kp"=25.0, "Ki"=2.0}], "Limits"={"StepSize"=0.0, "Max"=0.0, "Min"=0.0}, "Cutoffs"={"Middle"=0.0, "Close"=0.0}, "FFinfo"={"FF_m"=0.0, "FF_b"=0.0}}, {"Name"="Volt_Speed", "PI Far->Close"=[{"Slew"=200.0, "Kp"=0.75, "Ki"=0.0}, {"Slew"=6.0, "Kp"=0.5, "Ki"=0.01}, {"Slew"=0.003, "Kp"=5.0, "Ki"=3.0}], "Limits"={"StepSize"=0.0, "Max"=0.0, "Min"=0.0}, "Cutoffs"={"Middle"=0.0, "Close"=0.0}, "FFinfo"={"FF_m"=0.0, "FF_b"=0.0}}, {"Name"="Pres_Direct", "PI Far->Close"=[{"Slew"=25.0, "Kp"=0.4, "Ki"=0.0}, {"Slew"=2.0, "Kp"=35.0, "Ki"=0.3}, {"Slew"=0.1, "Kp"=35.0, "Ki"=0.3}], "Limits"={"StepSize"=0.0, "Max"=0.0, "Min"=0.0}, "Cutoffs"={"Middle"=0.0, "Close"=0.0}, "FFinfo"={"FF_m"=0.0, "FF_b"=0.0}}, {"Name"="Pres_Flow", "PI Far->Close"=[{"Slew"=65.0, "Kp"=-5.0, "Ki"=0.0}, {"Slew"=25.0, "Kp"=-25.0, "Ki"=-1.0}, {"Slew"=0.0, "Kp"=-250.0, "Ki"=-120.0}], "Limits"={"StepSize"=0.0, "Max"=0.0, "Min"=0.0}, "Cutoffs"={"Middle"=0.0, "Close"=0.0}, "FFinfo"={"FF_m"=0.0, "FF_b"=0.0}}, {"Name"="Pres_Speed", "PI Far->Close"=[{"Slew"=50.0, "Kp"=-100.0, "Ki"=-10.0}, {"Slew"=1.0, "Kp"=-50.0, "Ki"=-7.5}, {"Slew"=1.0, "Kp"=-50.0, "Ki"=-7.5}], "Limits"={"StepSize"=0.0, "Max"=0.0, "Min"=0.0}, "Cutoffs"={"Middle"=0.0, "Close"=0.0}, "FFinfo"={"FF_m"=0.0, "FF_b"=0.0}}, {"Name"="CMD_Direct", "PI Far->Close"=[{"Slew"=1.0, "Kp"=1.0, "Ki"=0.1}, {"Slew"=1.0, "Kp"=1.0, "Ki"=0.1}, {"Slew"=1.0, "Kp"=1.0, "Ki"=0.1}], "Limits"={"StepSize"=0.0, "Max"=0.0, "Min"=0.0}, "Cutoffs"={"Middle"=0.0, "Close"=0.0}, "FFinfo"={"FF_m"=0.0, "FF_b"=0.0}}, {"Name"="CMD_Flow", "PI Far->Close"=[{"Slew"=650.0, "Kp"=10.0, "Ki"=1.0}, {"Slew"=50.0, "Kp"=100.0, "Ki"=2.0}, {"Slew"=10.0, "Kp"=140.0, "Ki"=5.0}], "Limits"={"StepSize"=0.0, "Max"=0.0, "Min"=0.0}, "Cutoffs"={"Middle"=0.0, "Close"=0.0}, "FFinfo"={"FF_m"=0.0, "FF_b"=0.0}}, {"Name"="CMD_Speed", "PI Far->Close"=[{"Slew"=999999.0, "Kp"=0.0, "Ki"=0.0}, {"Slew"=999999.0, "Kp"=0.0, "Ki"=0.0}, {"Slew"=999999.0, "Kp"=0.0, "Ki"=0.15}], "Limits"={"StepSize"=0.0, "Max"=0.0, "Min"=0.0}, "Cutoffs"={"Middle"=0.0, "Close"=0.0}, "FFinfo"={"FF_m"=0.0, "FF_b"=0.0}}] ("ControlArray")
  (unwired) u32 16744703
  (unwired) u32 6618880
  (unwired) u32 9567230
  (unwired) u32 16777226
  (unwired) u32 16776960
  (unwired) u32 16776960
  (unwired) u32 255
  (unwired) u32 32768
  (unwired) u32 16711680
  w8 = T1 {"Para1"=0, "SP1"=0.0, "Para2"=1, "SP2"=0.0, "Para3"=4, "SP3"=10.0}  # CommandCluster
  w27 = T2 {"Pump Voltage (V)"=0.0, "Pump Current (Arms)"=0.0, "Pressure (kPA)"=0.0, "Flow (L/H)"=0.0, "Controller Voltage (V)"=0.0, "Controller Current (A)"=0.0, "Fuel Temp (C)"=0.0, "Speed (RPM)"=0.0, "Efficiency (%)"=0.0, "Stabilized?"=FALSE, "Controller CMD"=0.0}  # InstDataCluster
  w6 = 4000.0  # CMD Scaler
  w7 = T2 {"Pump Voltage (V)"=0.0, "Pump Current (Arms)"=0.0, "Pressure (kPA)"=0.0, "Flow (L/H)"=0.0, "Controller Voltage (V)"=0.0, "Controller Current (A)"=0.0, "Fuel Temp (C)"=0.0, "Speed (RPM)"=0.0, "Efficiency (%)"=0.0, "Stabilized?"=FALSE, "Controller CMD"=0.0}  # AveDataCluster
  w9 = T9 {"Stability Reads"=0, "Stability1"=0, "Stability2"=0, "Stability3"=0}  # StabilityCluster
  w10 = FALSE  # PS Enable
  w11 = dbl[][] []  # Cal Coeffs
  w12 = enum16{"Pump", "Controller"}."Controller"  # EnumV
  w16 = 0.0  # PC Data Timer
  w17 = 0.0  # PC Data Rate (sec)
  w21 = FALSE  # Deadhead?
  w22 = dbl[] []  # Tolerances
  w23 = Event_Mode."Init" ("Mode")
  w26 = u32 0  # PWM Period (ticks)
  w34 = 0.0  # FPGA Data Timer
  w35 = 0.0  # FPGA Data Rate (sec)
  w36 = 0.0  # PI Timer
  w37 = 0.0  # PI Rate (sec)
  # "Any StepSize, Max, Min, or IndMin\nchanges to a controller has to be\nimplemented in the Controller List"
  # "Any changes to Controller List here have\nto be applied to the controller list in PC also"
  # "Backup"
  # "Trace Engine won't work because of\nProperty Nodes"
  # "Controller List is now stored in main bundle\nand any updates need to happen there"
  # "CMD"
  # "-Tol"
  # "+Tol"
  # "AveS"
  # "Speed"
  # "AveF"
  # "Flow"
  # "AveV"
  # "Volt"
  # "Inside the Cal File I would like to start including Date Cal Completed and Due Date for Next Cal, I can then cast that down to PC to include in every data file"
  # "V\nP\nF\nS\nCMD"
  # "0 - Voltage\n1 - Pressure\n2 - Flow\n3 - Speed\n4 - Deadhead"
  n1 = local write "CmdCluster"(w8) -> ()
  n2 = Bundle("CommandCluster"=w8, "Deadhead?"=w21, "PI Rate (sec)"=w37, "PI Timer"=w36, "FPGA Data Rate (sec)"=w35, "FPGA Data Timer"=w34, "PC Data Rate (sec)"=w17, "PC Data Timer"=w16, "InstDataCluster"=w27, "Controller"=w4, "PWM Period (ticks)"=w26, "Tolerances"=w22, "Cal Coeffs"=w11, "EnumV"=w12, "PS Enable"=w10, "StabilityCluster"=w9, "AveDataCluster"=w7, "CMD Scaler"=w6, "ControlArray"=w3, "Controller List"=w2, "VandPLimit"=w5) -> (w38:T13)  [unwired: 1 in]
  n3 = call "RT Send Event.vi"("RTsend/PCrecv CMD"=RTsend_PCrecv_CMD."Data", "Mode"=w23) -> ("Error Out"=w33:errorcluster)  [unwired: 12 in, 1 out]
  n4 = call "RT Recv Event.vi"("Mode"=w23, "Error In"=w33) -> ("Error Out"=w32:errorcluster)  [unwired: 12 in, 1 out]
  n5 = call "RT Recv Event.vi"("Mode"=Event_Mode."Get", "Error In"=w32) -> ("PCsend/RTrecv Cluster"=w30:refnum<user-event>, "Error Out"=w31:errorcluster)  [unwired: 12 in]
  n6 = register-events(error in=w31, w30) -> (reference out=w29:refnum<event-registration>, error out=w25:errorcluster)  [unwired: 1 in]
  n7 = control-ref of="TraceCluster"() -> (w14:refnum<vi>)
  n8 = xnode ("Open FPGA VI Reference")("resource name"=tag "RIO0") -> ("FPGA VI Reference Out"=w40:refnum<k20>)  [unwired: 1 in, 1 out]
  n9 = control-ref of="Cal Coeffs"() -> (w13:refnum<vi>)
  n10 = Generate Occurrence() -> (w15:refnum<k4>)
  n11 = disable-structure shown="Disabled" {
    disable-tunnel: w40 -> [w43 _]
    disable-tunnel: w14 -> [w42 _]
    disable-tunnel: w13 -> [w41 _]
    frame Disabled {
      n12 = call "Trace Engine.vi"("FPGA VI Reference"=w43, "Arr Refnum"=w41, "TraceCluster"=w42) -> ()  [unwired: 13 in]
    }
    frame Enabled {
    }
  }
  n13 = while {
    shift-right: [w51] -> _
    shift-left: string[] ["Init"] -> [w55]
    shift-right: [w48] -> _
    shift-left: w38 -> [w50]
    shift-right: [w46] -> _
    shift-left: w40 -> [w47]
    tunnel: w29 -> [w45]
    tunnel: w15 -> [w44]
    stop <- w49 stop-if-true
    n14 = Delete From Array(array=w55, index=0) -> (deleted portion=w52:string, array with subset deleted=w53:string[])  [unwired: 1 in]
    n15 = case shown="\"Init\"" w52 {
      tunnel: w53 -> [w98 w157 w399 w477 w555 w568 w581]
      tunnel: [w97 w153 w399 w495 w555 w568 w581] -> w51
      tunnel: w50 -> [w89 w156 w370 w521 w552 w560 w572]
      tunnel: [_ FALSE _ _ _ _ _] -> w49
      tunnel: [w99 w154 w397 w520 w552 w567 w580] -> w48
      tunnel: w47 -> [w112 w151 w398 w514 w554 w569 w582]
      tunnel: [w100 w150 w398 w514 w553 w569 w582] -> w46
      tunnel: w45 -> [_ w149 _ _ _ _ _]
      tunnel: w44 -> [w96 _ _ _ _ _ _]
      frame "Init" {
        w73 = fxp<+/-,24,7> 0.0 ("Threshold level")
        w72 = 2 ("CommSegs")
        w71 = u32 400000 ("PWM Period (ticks)")
        w88 = dbl[] [0.2, 3.0, 3.0, 15.0, 5.0]
        w95 = FALSE ("PS Enable")
        w83 = 0.1 ("PI Timer")
        # "Vtol\nPtol\nFtol\nRPMtol\nTs"
        # "This is 10.30.189.0"
        n16 = xnode "Invoke Method"("FPGA VI Reference In"=w112) -> ("FPGA VI Reference Out"=w81:refnum<k20>, "error out"=w80:errorcluster)  [unwired: 1 in]
        n17 = local write "Hysteresis"(fxp<+,10,6> 0.0625 ("Hysteresis")) -> ()
        n18 = local write "PWM Period (ticks)"(w71) -> ()
        n19 = local write "CommSegs"(w72) -> ()
        n20 = local write "Threshold"(w73) -> ()
        n21 = local write "ave pts"(10 ("ave pts")) -> ()
        n22 = disable-structure shown="Enabled" {
          disable-tunnel: w81 -> [w124 w132]
          disable-tunnel: w80 -> [w123 w131]
          disable-tunnel: [w122 w130] -> w79
          disable-tunnel: [w121 w129] -> w78
          disable-tunnel: "Count 1(uS)" -> [w120 w128]
          disable-tunnel: "Count 2(uS)" -> [w119 w127]
          disable-tunnel: TRUE ("BL Threshold") -> [w118 _]
          disable-tunnel: 40000 ("PWM Duty") -> [w117 w126]
          disable-tunnel: w73 -> [w116 _]
          disable-tunnel: w72 -> [w115 _]
          disable-tunnel: w71 -> [w114 w125]
          frame Disabled {
            n23 = xnode "Read/Write Control"("FPGA VI Reference In"=w124, "error in"=w123, "Count 1(uS)"=w120, "Count 2(uS)"=w119, "Set Threshold"=w118, "PWM Duty"=w117, "PWM Period (ticks)"=w114, "CommSegs"=w115, "Threshold level"=w116) -> ("FPGA VI Reference Out"=w121:refnum<k20>, "error out"=w122:errorcluster)
          }
          frame Enabled {
            n24 = xnode "Read/Write Control"("FPGA VI Reference In"=w132, "error in"=w131, "Count 1(uS)"=w128, "Count 2(uS)"=w127, "PWM Duty"=w126, "PWM Period (ticks)"=w125) -> ("FPGA VI Reference Out"=w129:refnum<k20>, "error out"=w130:errorcluster)
          }
        }
        n25 = case shown="\"Page 1\", Default" "GraphTab" {
          frame "Page 1", Default {
            n26 = control-ref of="WFG1"() -> (w136:refnum<vi>)
            n27 = control-ref of="WFG2"() -> (w137:refnum<vi>)
            n28 = control-ref of="WFG3"() -> (w139:refnum<vi>)
            n29 = Build Array(w136, w137, w139) -> (w138:refnum<vi>[])
            n30 = call "Graph Handler.vi"("WF Ref Array"=w138, "State"="Init", "ChSize"=150, "NumCh"=27) -> ()  [unwired: 12 in]
          }
          frame "Page 2" {
            n31 = control-ref of="WFG4"() -> (w144:refnum<vi>)
            n32 = control-ref of="WFG5"() -> (w143:refnum<vi>)
            n33 = control-ref of="WFG6"() -> (w142:refnum<vi>)
            n34 = Build Array(w144, w143, w142) -> (w141:refnum<vi>[])
            n35 = call "Second Graph Handler.vi"("WF Ref Array"=w141, "State"="Init") -> ()  [unwired: 14 in]
          }
        }
        n36 = String To IP() -> (0:w109:u32)  [unwired: 1 in]
        n37 = Subtract(x=w109, y=u32 169786624) -> (x-y=w108:u32)
        n38 = xnode "Invoke Method"("FPGA VI Reference In"=w78, "error in"=w79) -> ("FPGA VI Reference Out"=w102:refnum<k20>)  [unwired: 1 in, 1 out]
        n39 = Number To Decimal String(number=w108) -> (decimal integer string=w107:string)  [unwired: 1 in]
        n40 = local write "Controller Name"(Controller_Names."Kuhnke" ("Controller Name")) -> ()
        n41 = local write "PS Enable"(w95) -> ()
        n42 = local write "Deadhead?"(w95) -> ()
        n43 = Concatenate Strings("/c/" ("string"), w107, ".cal" ("string")) -> (w104:string)
        n44 = String To Path(string=w104) -> (path=w103:path)
        n45 = Unbundle By Name(w89) -> ("ControlArray"=w68:T3)
        n46 = call "Get Cal Coefficients.vi"("Path"=w103) -> ("Error Out"=w92:errorcluster, "Dates"=w93:dbl[], "Cal Coefficients"=w94:dbl[][])  [unwired: 8 in]
        n47 = call <vilib>:"Clear Errors.vi"("error in (no error)"=w92) -> ("error out"=w66:errorcluster)  [unwired: 6 in]
        n48 = call "NEW RW Controls INI.vi"("Filepath"=path "c:/NEW Controls.ini", "Read (F)"=TRUE, "ControlArray In"=w68, "Error In"=w66) -> ("ControlArray Out"=w64:T3, "Error Out"=w58:errorcluster)  [unwired: 10 in]
        n49 = Index Array(array=w88, index=4) -> (element=w84:dbl)
        n50 = Divide(x=w84, y=w83) -> (x/y=w86:dbl)
        n51 = Array Max & Min(array=w93) -> (min value=→"PrevCalDate":dbl)  [unwired: 3 out]
        n52 = local write "Cal Coeffs"(w94) -> ()
        n53 = call "RW Controller Settings.vi"("Filepath"=path "c:/Controller Settings.ini", "Read (F)"=TRUE, "Controller Name"="Kuhnke", "ControlArray In"=w64, "Error In"=w58) -> ("ControlArray Out"=w63:T3)  [unwired: 9 in, 1 out]
        n54 = Round Toward +Infinity(x=w86) -> (ceil(x): smallest int >= x=w85:dbl)
        n55 = Get Date/Time In Seconds() -> (seconds since 1Jan1904=w113:timestamp)
        n56 = local write "ControlArray"(w63) -> ()
        n57 = To Long Integer(number=w85) -> (32bit integer=w82:i32)
        n58 = To Double Precision Float(number=w113) -> (double precision float=w90:dbl)
        n59 = Bundle By Name(cluster=w89, "ControlArray"=w63, "PI Timer"=w90, "FPGA Data Timer"=w90, "PC Data Timer"=w90, "PI Rate (sec)"=w83, "FPGA Data Rate (sec)"=0.1 ("FPGA Data Timer"), "PC Data Rate (sec)"=0.33 ("PC Data Timer"), "Cal Coeffs"=w94, "Tolerances"=w88, "StabilityCluster.Stability Reads"=w82, "StabilityCluster.Stability1"=w82, "StabilityCluster.Stability2"=w82, "StabilityCluster.Stability3"=w82) -> (w101:T13)
        n60 = flat-sequence {
          tunnel: w102 -> [w148]
          tunnel: w101 -> [w147]
          tunnel: [w148] -> w100
          tunnel: [w147] -> w99
          tunnel: w98 -> [w146]
          tunnel: [w146] -> w97
          tunnel: w96 -> [w145]
          frame #0 {
            n61 = Set Occurrence(w145) -> ()
          }
        }
      }
      frame "***MAIN***", Default {
        n62 = event shown="[1] <PCsend/RTrecv Cluster>: User Event" {
          selector: w149 -> [_ _]
          dyn-events: _ -> [_ _]
          timeout: 10 -> [_ _]
          tunnel: w157 -> [w171 w229]
          tunnel: w156 -> [w169 w232]
          tunnel: [w164 w231] -> w154
          tunnel: [w159 w228] -> w153
          tunnel: w151 -> [w179 w225]
          tunnel: [w179 w227] -> w150
          event Timeout {
            # "Was originally just going to read the FPGA\nand handle the PIs in the same case.\nRealized might want to run the PI slower\nthan I am updating the PC so seperated\nthe cases"
            # "FPGA Data Rate 0.1\nPI Rate 0.1\nPC Data Rate 0.33"
            # "_______________           _"
            n63 = event-data() -> ()  [unwired: 1 in, 3 out]
            n64 = Unbundle By Name(w169) -> ("PC Data Timer"=w177:dbl, "PC Data Rate (sec)"=w175:dbl, "FPGA Data Timer"=w173:dbl, "FPGA Data Rate (sec)"=w172:dbl, "PI Timer"=w166:dbl, "PI Rate (sec)"=w167:dbl)
            n65 = Get Date/Time In Seconds() -> (seconds since 1Jan1904=w178:timestamp)
            n66 = To Double Precision Float(number=w178) -> (double precision float=w165:dbl)
            n67 = Subtract(x=w165, y=w177) -> (x-y=w176:dbl)
            n68 = Subtract(x=w165, y=w173) -> (x-y=w174:dbl)
            n69 = Subtract(x=w165, y=w166) -> (x-y=w168:dbl)
            n70 = Greater?(x=w176, y=w175) -> (0:w170:bool)
            n71 = Greater?(x=w174, y=w172) -> (0:w161:bool)
            n72 = Greater?(x=w168, y=w167) -> (0:w163:bool)
            n73 = case shown="True" w163 {
              tunnel: w171 -> [w190 w194]
              tunnel: [w190 w193] -> w162
              frame False {
              }
              frame True {
                n74 = Insert Into Array(array=w194, index=0, new element=string[] ["PI Controller"]) -> (w193:string[])
              }
            }
            n75 = case shown="True" w170 {
              tunnel: [w195 w214] -> w164
              tunnel: w165 -> [_ w213]
              tunnel: w169 -> [w195 w199]
              tunnel: [FALSE "SaveConfig"] -> w158
              frame False {
              }
              frame True {
                n76 = flat-sequence {
                  tunnel: ["Cal Coeffs"] -> w209
                  tunnel: ["PS Enable"] -> w208
                  tunnel: ["Deadhead?"] -> w207
                  tunnel: ["EnumV"] -> w206
                  tunnel: ["CmdCluster"] -> w205
                  tunnel: ["ControlArray"] -> w198
                  frame #0 {
                    n77 = local read "CmdCluster"() -> (w215:T1)
                    n78 = Select(t="CMD to Load", s="Load Cmd", f=w215) -> (s? t:f=w216:T1)
                    n79 = local write "CmdCluster"(w216) -> ()
                  }
                  frame #1 {
                  }
                }
                n80 = Unbundle By Name(w199) -> ("AveDataCluster"=w201:T2)
                n81 = Flatten To String(anything=w201) -> (data string=w200:string)  [unwired: 3 in, 2 out]
                n82 = Bundle(cluster=T14 {"Command"="", "FlattenedData"=""}, "Command"="Data", "FlattenedData"=w200) -> (w203:T14)
                n83 = Flatten To String(anything=w203) -> (data string=w211:string)  [unwired: 3 in, 2 out]
                n84 = Bundle By Name(cluster=w199, "PC Data Timer"=w213, "Cal Coeffs"=w209, "CommandCluster"=w205, "PS Enable"=w208, "Deadhead?"=w207, "EnumV"=w206, "ControlArray"=w198) -> (w214:T13)
                n85 = call "RT Send Event.vi"("RTsend/PCrecv CMD"=RTsend_PCrecv_CMD."Data" ("RT Send Command"), "Mode"=Event_Mode."Set", "Flattened Data"=w211) -> ()  [unwired: 11 in, 2 out]
              }
            }
            n86 = case shown="True" w161 {
              tunnel: w162 -> [w185 w189]
              tunnel: [w185 w188] -> w160
              frame False {
              }
              frame True {
                n87 = Insert Into Array(array=w189, index=0, new element=string[] ["Read Data"]) -> (w188:string[])
              }
            }
            n88 = case shown="True" w158 {
              tunnel: w160 -> [w180 w184]
              tunnel: [w180 w183] -> w159
              frame False {
              }
              frame True {
                n89 = Insert Into Array(array=w184, index=0, new element=string[] ["Save Config"]) -> (w183:string[])
              }
            }
          }
          event User Event {
            n90 = event-data() -> ("PCsend/RTrecv CMD"=w226:T16, "Flattened Data"=w230:string)  [unwired: 1 in]
            n91 = case shown="\"Controller\"" w226 {
              tunnel: w232 -> [w235 w237 w240 w253 w290 w317 w331 w335 w357 w365]
              tunnel: [w235 w237 w240 w252 w303 w316 w331 w349 w357 w364] -> w231
              tunnel: w230 -> [_ _ _ w255 w302 w319 _ w348 _ w363]
              tunnel: w229 -> [w234 w236 w239 w256 w281 w315 w330 w333 w353 w360]
              tunnel: [w234 w236 w239 w256 w280 w315 w330 w333 w353 w360] -> w228
              tunnel: w225 -> [w233 w238 w241 w257 w298 w321 w332 w347 w356 w366]
              tunnel: [w233 w238 w241 w257 w298 w320 w332 w347 w355 w366] -> w227
              frame Default {
                # "Shouldn't ever get here\nwhich would mean something is not setup correctly"
              }
              frame "ConnSettings" {
              }
              frame "Connect" {
              }
              frame "CMD" {
                w254 = T1 {"Para1"=0, "SP1"=0.0, "Para2"=0, "SP2"=0.0, "Para3"=0, "SP3"=0.0}  # CommandCluster
                # "In PC I am sending the CmdCluster over as it appears to the user\n\nHere I am taking care of adjusting it to handle using the correct\n    controls to reach the parameters"
                n92 = Unflatten From String(type=w254, binary string=w255) -> (value=w248:T1)  [unwired: 3 in, 2 out]
                n93 = Unbundle By Name(w248) -> ("Para1"=w242:i32, "SP1"=w245:dbl, "Para2"=w243:i32, "SP2"=w244:dbl)
                n94 = Equal To 0?(x=w242) -> (x = 0?=w246:bool)
                n95 = case shown="False" w246 {
                  tunnel: w248 -> [w263 w264]
                  tunnel: [w262 w264] -> w247
                  tunnel: w242 -> [w261 _]
                  tunnel: w245 -> [w260 _]
                  tunnel: w243 -> [w259 _]
                  tunnel: w244 -> [w258 _]
                  frame False {
                    n96 = Bundle By Name(cluster=w263, "Para2"=w261, "SP2"=w260, "Para1"=w259, "SP1"=w258) -> (w262:T1)
                  }
                  frame True {
                  }
                }
                n97 = Unbundle By Name(w247) -> ("Para2"=w251:i32)
                n98 = Equal?(x=w251, y=4) -> (x = y?=w249:bool)
                n99 = local write "CmdCluster"(w247) -> ()
                n100 = Bundle By Name(cluster=w253, "CommandCluster"=w247, "Deadhead?"=w249) -> (w252:T13)
                n101 = local write "Deadhead?"(w249) -> ()
              }
              frame "Controller" {
                w301 = 0  # Controller Index
                # "Don't need to know PWM?\nbecause that is handled by\nonly CAN controllers having\na subVI in the bottom loop"
                n102 = Unbundle By Name(w290) -> ("Controller List"=w266:T6, "PS Enable"=w289:bool, "ControlArray"=w271:T3)
                n103 = Unflatten From String(type=w301, binary string=w302) -> (value=w300:i32)  [unwired: 3 in, 2 out]
                n104 = Index Array(array=w266, index=w300) -> (element=w299:T7)
                n105 = Unbundle By Name(w299) -> ("Controller?"=w277:bool, "Controller Name"=→"Controller Name":T5, "CommSeg"=w274:i32, "Solenoid Stop?"=w287:bool, "Frequency"=w286:i32, "Stop Command"=w276:dbl, "Command Step"=w270:dbl, "High Command"=w269:dbl, "Low Command"=w268:dbl, "Indirect Nonzero CMD"=w265:dbl)
                n106 = Insert Into Array(array=w281, index=0, new element=string[] ["Load Controller Settings", "Save Config"]) -> (w280:string[])
                n107 = call "NEW Set Controller Limits.vi"("IndMin"=w265, "Min"=w268, "Max"=w269, "StepSize"=w270, "ControlArray In"=w271) -> ("ControlArray Out"=w267:T3)  [unwired: 10 in]
                n108 = Not(x=w277) -> (.not. x?=w285:bool)
                n109 = Divide(x=40000000.0 ("PWM Period (Ticks)"), y=w286) -> (x/y=w293:dbl)
                n110 = Boolean To (0,1)(Boolean=w285) -> (0, 1=w284:i16)
                n111 = Divide(x=w293, y=100.0 ("PWM Period (Ticks)")) -> (x/y=w275:dbl)
                n112 = To Unsigned Long Integer(number=w293) -> (unsigned 32bit integer=w295:u32)
                "PWM Period (ticks)" <- w295
                n113 = local write "EnumV"(w284) -> ()
                n114 = Equal?(x=w274, y=2) -> (x = y?=w273:bool)
                n115 = Select(t=FALSE, s=w287, f=w289) -> (s? t:f=w282:bool)
                n116 = Multiply(x=w275, y=w276) -> (x*y=w292:dbl)
                n117 = Not(x=w273) -> (.not. x?=w272:bool)
                n118 = To Long Integer(number=w292) -> (32bit integer=w291:i32)
                n119 = disable-structure shown="Enabled" {
                  disable-tunnel: w298 -> [w309 w313]
                  disable-tunnel: w295 -> [w308 w312]
                  disable-tunnel: w291 -> [w307 w311]
                  disable-tunnel: w274 -> [w306 _]
                  disable-tunnel: w273 -> [w305 _]
                  disable-tunnel: w272 -> [w304 w310]
                  frame Disabled {
                    n120 = xnode "Read/Write Control"("FPGA VI Reference In"=w309, "CommSegs"=w306, "Set Threshold"=w305, "PWM Duty"=w307, "PWM Period (ticks)"=w308, "Brushed Speed"=w304) -> ()  [unwired: 1 in, 2 out]
                  }
                  frame Enabled {
                    n121 = xnode "Read/Write Control"("FPGA VI Reference In"=w313, "PWM Duty"=w311, "PWM Period (ticks)"=w312, "Brushed Speed"=w310) -> ()  [unwired: 1 in, 2 out]
                  }
                }
                n122 = Bundle By Name(cluster=w290, "CMD Scaler"=w275, "Controller"=w299, "EnumV"=w284, "PWM Period (ticks)"=w295, "ControlArray"=w267, "PS Enable"=w282) -> (w303:T13)
                n123 = local write "PS Enable"(w282) -> ()
                n124 = local write "ControlArray"(w267) -> ()
                n125 = local write "Brushed Speed"(w272) -> ()
                n126 = local write "CommSegs"(w274) -> ()
              }
              frame "PSenable" {
                n127 = Unflatten From String(type=FALSE, binary string=w319) -> (value=w314:bool)  [unwired: 3 in, 2 out]
                n128 = Bundle By Name(cluster=w317, "PS Enable"=w314) -> (w316:T13)
                n129 = xnode "Read/Write Control"("FPGA VI Reference In"=w321, "PSenable"=w314) -> ("FPGA VI Reference Out"=w320:refnum<k20>)  [unwired: 1 in, 1 out]
                n130 = local write "PS Enable"(w314) -> ()
              }
              frame "ReqCalDate" {
                n131 = local read "PrevCalDate"() -> (w322:dbl)
                n132 = Flatten To String(anything=w322) -> (data string=w323:string)  [unwired: 3 in, 2 out]
                n133 = Bundle(cluster=T14 {"Command"="", "FlattenedData"=""}, "Command"="CalFileDate", "FlattenedData"=w323) -> (w325:T14)
                n134 = Flatten To String(anything=w325) -> (data string=w328:string)  [unwired: 3 in, 2 out]
                n135 = call "RT Send Event.vi"("RTsend/PCrecv CMD"=RTsend_PCrecv_CMD."CalFileDate" ("RT Send Command"), "Mode"=Event_Mode."Set", "Flattened Data"=w328) -> ()  [unwired: 11 in, 2 out]
              }
              frame "Tolerances" {
                w340 = T17 {"Voltage Tolerances"=0.0, "Pressure Tolerances"=0.0, "Flow Tolerances"=0.0, "Speed Tolerances"=0.0, "Stable Count (sec)"=0.0}  # Stability Cluster
                n136 = Unbundle By Name(w335) -> ("PI Rate (sec)"=w339:dbl)
                n137 = Unflatten From String(type=w340, binary string=w348) -> (value=w346:T17)  [unwired: 3 in, 2 out]
                n138 = Unbundle By Name(w346) -> ("Voltage Tolerances"=w345:dbl, "Pressure Tolerances"=w344:dbl, "Flow Tolerances"=w343:dbl, "Speed Tolerances"=w342:dbl, "Stable Count (sec)"=w336:dbl)
                n139 = Divide(x=w336, y=w339) -> (x/y=w338:dbl)
                n140 = Build Array(w345, w344, w343, w342) -> (w341:dbl[])
                n141 = Round Toward +Infinity(x=w338) -> (ceil(x): smallest int >= x=w337:dbl)
                n142 = To Long Integer(number=w337) -> (32bit integer=w334:i32)
                n143 = Bundle By Name(cluster=w335, "Tolerances"=w341, "StabilityCluster.Stability Reads"=w334, "StabilityCluster.Stability1"=w334, "StabilityCluster.Stability2"=w334, "StabilityCluster.Stability3"=w334) -> (w349:T13)
              }
              frame "Stable Trigger" {
                n144 = xnode "Read/Write Control"("FPGA VI Reference In"=w356, "StableTrigger"=fxp<+/-,20,5> 5.0) -> ("FPGA VI Reference Out"=w351:refnum<k20>)  [unwired: 1 in, 1 out]
                n145 = flat-sequence {
                  tunnel: w351 -> [w359]
                  tunnel: [w359] -> w350
                  frame #0 {
                    n146 = Wait (ms)(milliseconds to wait=u32 10) -> ()  [unwired: 1 out]
                  }
                }
                n147 = xnode "Read/Write Control"("FPGA VI Reference In"=w350, "StableTrigger"=fxp<+/-,20,5> 0.0) -> ("FPGA VI Reference Out"=w355:refnum<k20>)  [unwired: 1 in, 1 out]
              }
              frame "VPLimits" {
                n148 = Unflatten From String(type=dbl[] [], binary string=w363) -> (value=w361:dbl[])  [unwired: 3 in, 2 out]
                n149 = Bundle By Name(cluster=w365, "VandPLimit"=w361) -> (w364:T13)
              }
            }
          }
        }
      }
      frame "Read Data" {
        # "CommSeg is coming through as 2, 8, or 10"
        # "At a startup the first reading is saturation when controlling\nto speed with voltage that means the voltage is dropped to\ncompensate which then the pump just pulses on/off"
        # "Efficiency % = ( 36 * Pressure * Flow ) / ( Voltage * Current )"
        n150 = disable-structure shown="Enabled" {
          disable-tunnel: w398 -> [w409 w422 _]
          disable-tunnel: [w400 w410 w423] -> w373
          frame Enabled {
            n151 = xnode "Read/Write Control"("FPGA VI Reference In"=w409, "Hysteresis"="Hysteresis", "CtCuttoff"="CtCuttoff") -> ("DataCluster"=w408:T18)  [unwired: 1 in, 2 out]
            n152 = Cluster To Array(cluster=w408) -> (array=w405:fxp<+/-,25,15>[])
            n153 = local read "Speed"() -> (w403:dbl)
            n154 = To Double Precision Float(number=w405) -> (double precision float=w404:dbl[])
            n155 = Replace Array Subset(array=w404, new element=w403, index=7) -> (w400:dbl[])
            n156 = call "AI RT FIFO.vi"("Data IN"=w400, "Mode"=Stream_RT_FIFO_Mode."Write") -> ()  [unwired: 11 in, 3 out]
          }
          frame Disabled {
            n157 = xnode "Read/Write Control"("FPGA VI Reference In"=w422) -> ("DataCluster"=w421:T18, "Hysteresis"=w419:fxp<+,24,5>, "Set Threshold"=w418, "CommSegs"=w417, "Threshold level"=w416, "CtCuttoff"=w412:fxp<+,24,5>)  [unwired: 1 in, 2 out]
            n158 = Cluster To Array(cluster=w421) -> (array=w415:fxp<+/-,25,15>[])
            n159 = local read "Speed"() -> (w413:dbl)
            n160 = To Double Precision Float(number=w415) -> (double precision float=w414:dbl[])
            n161 = Replace Array Subset(array=w414, new element=w413, index=7) -> (w410:dbl[])
            n162 = call "AI RT FIFO.vi"("Data IN"=w410, "Mode"=Stream_RT_FIFO_Mode."Write") -> ()  [unwired: 11 in, 3 out]
          }
          frame Disabled {
            n163 = local read "output array"() -> (w423:dbl[])
          }
        }
        n164 = Unbundle By Name(w370) -> ("InstDataCluster"=w393:T2, "Cal Coeffs"=w372:dbl[][])  [unwired: 1 out]
        n165 = call "Calibration Applier.vi"("Cal Coefficients"=w372, "Data In"=w373) -> ("Data Cluster"=w371:T19)  [unwired: 13 in]
        n166 = Unbundle(w371) -> ("[0]"=w382:dbl, "[1]"=w383:dbl, "[2]"=w368:dbl, "[3]"=w377:dbl, "[4]"=w376:dbl, "[5]"=w375:dbl, "[6]"=w381:dbl, "[7]"=w378:dbl)
        n167 = feedback-in #1("ave pts") -> ()
        n168 = feedback #1("ave pts") -> (w391:i32)
        n169 = call "Efficiency Calculation.vi"("Current"=w375, "Voltage"=w376, "Flow"=w377, "Pressure"=w368) -> ("%Efficiency"=w374:dbl)  [unwired: 7 in]
        n170 = Not Equal?(x=w391, y="ave pts") -> (x != y?=w379:bool)
        n171 = call <vilib>:"Mean PtByPt.vi"("x"=w383, "sample length"="ave pts", "initialize"=w379) -> ("mean"=w386:dbl)  [unwired: 1 in, 1 out]
        n172 = call <vilib>:"Mean PtByPt.vi"("x"=w377, "sample length"="ave pts", "initialize"=w379) -> ("mean"=w385:dbl)  [unwired: 1 in, 1 out]
        n173 = call <vilib>:"Mean PtByPt.vi"("x"=w375, "sample length"="ave pts", "initialize"=w379) -> ("mean"=w367:dbl)  [unwired: 1 in, 1 out]
        n174 = call <vilib>:"Mean PtByPt.vi"("x"=w378, "sample length"="ave pts", "initialize"=w379) -> ("mean"=w384:dbl)  [unwired: 1 in, 1 out]
        n175 = call <vilib>:"Mean PtByPt.vi"("x"=w382, "sample length"="ave pts", "initialize"=w379) -> ("mean"=w387:dbl)  [unwired: 1 in, 1 out]
        n176 = call <vilib>:"Mean PtByPt.vi"("x"=w368, "sample length"="ave pts", "initialize"=w379) -> ("mean"=w369:dbl)  [unwired: 1 in, 1 out]
        n177 = call <vilib>:"Mean PtByPt.vi"("x"=w376, "sample length"="ave pts", "initialize"=w379) -> ("mean"=w388:dbl)  [unwired: 1 in, 1 out]
        n178 = call <vilib>:"Mean PtByPt.vi"("x"=w381, "sample length"="ave pts", "initialize"=w379) -> ("mean"=w389:dbl)  [unwired: 1 in, 1 out]
        n179 = call <vilib>:"Mean PtByPt.vi"("x"=w374, "sample length"="ave pts", "initialize"=w379) -> ("mean"=w390:dbl)  [unwired: 1 in, 1 out]
        n180 = Bundle By Name(cluster=w393, "Pump Voltage (V)"=w382, "Pump Current (Arms)"=w383, "Pressure (kPA)"=w368, "Flow (L/H)"=w377, "Controller Voltage (V)"=w376, "Controller Current (A)"=w375, "Fuel Temp (C)"=w381, "Speed (RPM)"=w378, "Efficiency (%)"=w374) -> (w396:T2)
        "Inst Data Cluster" <- w396
        n181 = Bundle By Name(cluster=w393, "Pump Voltage (V)"=w387, "Pump Current (Arms)"=w386, "Pressure (kPA)"=w369, "Flow (L/H)"=w385, "Controller Voltage (V)"=w388, "Controller Current (A)"=w367, "Fuel Temp (C)"=w389, "Speed (RPM)"=w384, "Efficiency (%)"=w390) -> (w392:T2)
        "Ave Data Cluster" <- w392
        n182 = Get Date/Time In Seconds() -> (seconds since 1Jan1904=w395:timestamp)
        n183 = To Double Precision Float(number=w395) -> (double precision float=w394:dbl)
        n184 = Bundle By Name(cluster=w370, "FPGA Data Timer"=w394, "InstDataCluster"=w396, "AveDataCluster"=w392) -> (w397:T13)
      }
      frame "PI Controller" {
        w489 = 149
        w512 = 0.0 ("lower limit")
        w519 = fxp<+/-,20,5> 0.0 ("VoltCtrl")
        # "Deadhead or Controller CMD (ie 4) will skip PID"
        # "Have to add controller?\nas an input and adapt\nthe cmd vi\n\nfor third PI"
        n185 = Unbundle By Name(w521) -> ("Controller.Stop Command"=w446:dbl, "ControlArray"=w445:T3, "InstDataCluster"=w503:T2, "AveDataCluster"=w502:T2, "InstDataCluster.Controller Voltage (V)"=w443:dbl, "AveDataCluster.Controller Voltage (V)"=w442:dbl, "Tolerances"=w452:dbl[], "CommandCluster"=w426:T1, "StabilityCluster"=w465:T9, "Controller.Controller?"=w450:bool, "Controller.PWM?"=w506:bool, "CMD Scaler"=w447:dbl, "Deadhead?"=w499:bool, "PS Enable"=w482:bool, "InstDataCluster.Pressure (kPA)"=w476:dbl, "AveDataCluster.Pressure (kPA)"=w475:dbl, "InstDataCluster.Controller CMD"=w473:dbl, "AveDataCluster.Controller CMD"=w472:dbl, "InstDataCluster.Flow (L/H)"=w481:dbl, "AveDataCluster.Flow (L/H)"=w480:dbl, "InstDataCluster.Speed (RPM)"=w479:dbl, "AveDataCluster.Speed (RPM)"=w478:dbl, "VandPLimit"=w425:dbl[])
        n186 = call "Data Cluster to Feedback Array.vi"("AveDataCluster"=w502, "InstDataCluster"=w503) -> ("Ave FB"=w451:dbl[], "Inst FB"=w454:dbl[])
        n187 = Build Array(w476, w475) -> (w441:dbl[])
        n188 = Build Array(w473, w472) -> (w466:dbl[])
        n189 = Build Array(w481, w480, w479, w478) -> (w440:dbl[])
        n190 = call "NEWEST PI_0.vi"("ControlArray"=w445, "CommandCluster"=w426, "Run?"=TRUE, "Feedback"=w454, "VandPLimits"=w425, "Stability In"=w465, "Tolerances"=w452, "Controller?"=w450, "Ave Feedback"=w451) -> ("PIdata"=w464:dbl[], "Output"=w462:dbl, "Stable?"=w461:bool, "Stability Out"=w455:T9)  [unwired: 3 in]
        n191 = Not(x=w499) -> (.not. x?=w456:bool)
        n192 = call "NEWEST PI_1.vi"("ControlArray"=w445, "CommandCluster"=w426, "Run?"=w456, "Feedback"=w454, "VandPLimits"=w425, "Stability In"=w455, "Tolerances"=w452, "Controller?"=w450, "Ave Feedback"=w451) -> ("PIdata"=w457:dbl[], "Output"=w449:dbl, "Stable?"=w448:bool, "Stability Out"=w453:T9)  [unwired: 3 in]
        n193 = call "NEWEST PI_2.vi"("ControlArray"=w445, "Stop CMD"=w446, "CommandCluster"=w426, "Run?"=w450, "Feedback"=w454, "Stability In"=w453, "Tolerances"=w452, "Controller?"=w450, "Ave Feedback"=w451) -> ("PIdata"=w458:dbl[], "Output"=w424:dbl, "Stable?"=w459:bool, "Stability Out"=w460:T9)  [unwired: 3 in]
        n194 = call "Stability Timer.vi"("Stable 3"=w459, "Stable 2"=w448, "CommandCluster"=w426, "Stable"=w461) -> ("time 3"=→"time 3":dbl, "time 2"=→"time 2":dbl, "time"=→"time":dbl, "CMDchange"=w484:bool)  [unwired: 4 in]
        n195 = Index Array(array=w464) -> (element #1=w432:dbl, element #2=w431:dbl, element #3=w434:dbl, element #4=w435:dbl)  [unwired: 4 in]
        n196 = Index Array(array=w457) -> (element #1=w430:dbl, element #2=w429:dbl, element #3=w436:dbl, element #4=w437:dbl)  [unwired: 4 in]
        n197 = Index Array(array=w458) -> (element #1=w428:dbl, element #2=w427:dbl, element #3=w438:dbl, element #4=w439:dbl)  [unwired: 4 in]
        n198 = Select(t="VDirect", s="DirectV?", f=w462) -> (s? t:f=w509:dbl)
        n199 = Select(t="PresDirect", s="DirectPres?", f=w449) -> (s? t:f=w508:dbl)
        n200 = In Range and Coerce(upper limit=10.0, x=w509, lower limit=w512) -> (coerced(x)=w471:dbl)  [unwired: 1 out]
        "VSig" <- w471
        n201 = In Range and Coerce(upper limit=5.0, x=w508, lower limit=w512) -> (coerced(x)=w474:dbl)  [unwired: 1 out]
        "PresSig" <- w474
        n202 = Build Array (concatenate)(w466, w440, w438, w439, w424) -> (w468:dbl[])
        n203 = Build Array (concatenate)(w441, w440, w436, w437, w474) -> (w469:dbl[])
        n204 = feedback #2(w489) -> (w490:i32)
        n205 = Select(t=w489, s=w484, f=w490) -> (s? t:f=w494:i32)
        n206 = Decrement(x=w494) -> (x-1=w493:i32)
        n207 = Less Than 0?(x=w493) -> (x < 0?=w486:bool)
        n208 = Build Array (concatenate)(w443, w442, w440, w434, w435, w471) -> (w470:dbl[])
        n209 = Compound Arithmetic op=AND(w461, w448, w459) -> (w496:bool)
        n210 = feedback-in #3(w496) -> ()
        n211 = feedback #3(w496) -> (w498:bool)
        n212 = Not Equal?(x=w498, y=w496) -> (x != y?=w497:bool)
        n213 = case shown="True" w497 {
          tunnel: w477 -> [w527 w531]
          tunnel: [w527 w530] -> w495
          frame False {
          }
          frame True {
            n214 = Insert Into Array(array=w531, index=0, new element="Stable Trigger" ("new element/subarray")) -> (w530:string[])
          }
        }
        n215 = Not(x=w486) -> (.not. x?=w485:bool)
        n216 = Build Array (concatenate)(w470, w469, w468) -> (w467:dbl[])
        n217 = Select(t=0, s=w486, f=w493) -> (s? t:f=w491:i32)
        n218 = feedback-in #2(w491) -> ()
        n219 = To Fixed-Point(fixed-point type=w519, number=w471) -> (fixed-point=w517:fxp<+/-,20,5>)
        n220 = To Fixed-Point(fixed-point type=w519, number=w474) -> (fixed-point=w518:fxp<+/-,20,5>)
        n221 = Or(x=w485, y="constant update?") -> (x .or. y?=w487:bool)
        n222 = local read "GraphTab"() -> (w444:enum32{"Page 1", "Page 2"})
        n223 = Build Array (concatenate)(w443, w442, w441, w440, w424, w424, w434, w435, w436, w437, w438, w439, w432, w431, w430, w429, w428, w427) -> (w433:dbl[])
        n224 = case shown="False" w506 {
          tunnel: w514 -> [w535 w547]
          tunnel: w499 -> [w536 w546]
          tunnel: w517 -> [w537 w545]
          tunnel: w518 -> [w538 w544]
          tunnel: w482 -> [w533 w543]
          tunnel: w424 -> [w532 w540]
          tunnel: w447 -> [_ w539]
          frame False {
            n225 = To Unsigned Word Integer(number=w532) -> (unsigned 16bit integer=w534:u16)
            n226 = xnode "Read/Write Control"("FPGA VI Reference In"=w535, "Deadhead"=w536, "VoltCtrl"=w537, "PresCtrl"=w538, "PSenable"=w533) -> ()  [unwired: 1 in, 2 out]
            n227 = local write "CAN CMD"(w534) -> ()
          }
          frame True {
            n228 = Multiply(x=w539, y=w540) -> (x*y=w541:dbl)
            n229 = To Long Integer(number=w541) -> (32bit integer=w542:i32)
            n230 = xnode "Read/Write Control"("FPGA VI Reference In"=w547, "Deadhead"=w546, "VoltCtrl"=w545, "PresCtrl"=w544, "PSenable"=w543, "PWM Duty"=w542) -> ()  [unwired: 1 in, 2 out]
          }
        }
        n231 = Get Date/Time In Seconds() -> (seconds since 1Jan1904=w513:timestamp)
        n232 = To Double Precision Float(number=w513) -> (double precision float=w505:dbl)
        n233 = Bundle By Name(cluster=w521, "PI Timer"=w505, "InstDataCluster.Stabilized?"=w496, "InstDataCluster.Controller CMD"=w424, "StabilityCluster"=w460) -> (w520:T13)
        n234 = case shown="\"Page 2\"" w444 {
          tunnel: w487 -> [w524 w526]
          tunnel: w467 -> [_ w525]
          tunnel: w433 -> [w523 _]
          tunnel: w426 -> [w522 _]
          frame "Page 2" {
            n235 = call "Second Graph Handler.vi"("update?"=w524, "Data"=w523, "CommandCluster"=w522) -> ()  [unwired: 13 in]
          }
          frame "Page 1", Default {
            n236 = call "Graph Handler.vi"("update?"=w526, "Data"=w525) -> ()  [unwired: 14 in]
          }
        }
      }
      frame "Stable Trigger" {
        n237 = Unbundle By Name(w552) -> ("InstDataCluster.Stabilized?"=w551:bool)
        n238 = Select(t=fxp<+/-,20,5> 5.0 ("StableTrigger"), s=w551, f=fxp<+/-,20,5> 0.0 ("StableTrigger")) -> (s? t:f=w550:fxp<+/-,20,5>)
        n239 = xnode "Read/Write Control"("FPGA VI Reference In"=w554, "StableTrigger"=w550) -> ("FPGA VI Reference Out"=w553:refnum<k20>)  [unwired: 1 in, 1 out]
      }
      frame "Load Controller Settings" {
        n240 = Unbundle By Name(w560) -> ("Controller.Name"=w557:string, "ControlArray"=w564:T3)
        n241 = Unbundle By Name(w560) -> ("Controller.Command Step"=w563:dbl, "Controller.High Command"=w562:dbl, "Controller.Low Command"=w561:dbl, "Controller.Indirect Nonzero CMD"=w556:dbl)
        n242 = call "RW Controller Settings.vi"("Filepath"=path "c:/Controller Settings.ini", "Read (F)"=TRUE, "Controller Name"=w557, "ControlArray In"=w564) -> ("ControlArray Out"=w559:T3)  [unwired: 10 in, 1 out]
        n243 = call "NEW Set Controller Limits.vi"("IndMin"=w556, "Min"=w561, "Max"=w562, "StepSize"=w563, "ControlArray In"=w559) -> ("ControlArray Out"=w558:T3)  [unwired: 10 in]
        n244 = local write "ControlArray"(w558) -> ()
        n245 = Bundle By Name(cluster=w560, "ControlArray"=w558) -> (w567:T13)
      }
      frame "Save Config" {
        n246 = local read "ControlArray"() -> (w578:T3)
        n247 = Unbundle By Name(w572) -> ("Controller.Name"=w571:string)
        n248 = call "NEW RW Controls INI.vi"("Filepath"=path "c:/NEW Controls.ini", "ControlArray In"=w578) -> ("ControlArray Out"=w570:T3, "Error Out"=w577:errorcluster)  [unwired: 12 in]
        n249 = call <vilib>:"Clear Errors.vi"("error in (no error)"=w577) -> ("error out"=w576:errorcluster)  [unwired: 6 in]
        n250 = call "RW Controller Settings.vi"("Filepath"=path "c:/Controller Settings.ini", "Controller Name"=w571, "ControlArray In"=w570, "Error In"=w576) -> ("ControlArray Out"=w574:T3, "Error Out"=w575:errorcluster)  [unwired: 10 in]
        n251 = Bundle By Name(cluster=w572, "ControlArray"=w574) -> (w580:T13)
        n252 = call <vilib>:"Clear Errors.vi"("error in (no error)"=w575) -> ()  [unwired: 6 in, 1 out]
      }
    }
  }
  n253 = while {
    tunnel: w25 -> [w585]
    stop <- FALSE stop-if-true
    n254 = call <vilib>:"RT Get CPU Loads.vi"("error in (no error)"=w585) -> ("CPU loads"=w588:T20[])  [unwired: 9 in, 1 out]
    n255 = Index Array(array=w588) -> (element=w587:T20)  [unwired: 1 in]
    n256 = Unbundle By Name(w587) -> ("Total (%)"=→"Total (%)":dbl)
    n257 = Wait (ms)(milliseconds to wait=u32 500) -> ()  [unwired: 1 out]
  }
  n258 = disable-structure shown="Enabled" {
    disable-tunnel: w40 -> [w589 w619]
    disable-tunnel: dbl[] [0.0, 0.0, 0.0, 0.0, 0.0, 0.0, 0.0, 0.0, 0.0, 0.0] -> [_ w618]
    frame Enabled {
      n259 = while {
        tunnel: w589 -> [w604]
        shift-right: [w598] -> _
        shift-left: _ -> [w597]
        stop <- FALSE stop-if-true
        n260 = xnode "Read/Write Control"("FPGA VI Reference In"=w604) -> ("FPGA VI Reference Out"=w603:refnum<k20>, "Actual Loop Time"=→"Actual Loop Time":u32, "Actual Loop Time 2"=→"Actual Loop Time 2":u32)  [unwired: 1 in, 1 out]
        n261 = xnode "Invoke Method"("FPGA VI Reference In"=w603, "Number of Elements"=u32 0) -> ("FPGA VI Reference Out"=w606:refnum<k20>, "Elements Remaining"=w607:u32)  [unwired: 2 in, 2 out]
        n262 = Wait (ms)(milliseconds to wait=u32 100) -> ()  [unwired: 1 out]
        n263 = Get Date/Time In Seconds() -> (seconds since 1Jan1904=w600:timestamp)
        n264 = To Double Precision Float(number=w600) -> (double precision float=w598:dbl)
        n265 = xnode "Invoke Method"("FPGA VI Reference In"=w606, "Number of Elements"=w607) -> ("Data"=w596:fxp<+/-,24,5>[])  [unwired: 2 in, 3 out]
        n266 = Subtract(x=w598, y=w597) -> (x-y=→"Speed Loop Time":dbl)
        n267 = local read "CommSegs"() -> (w590:i32)
        n268 = To Double Precision Float(number=w596) -> (double precision float=w594:dbl[])
        n269 = case shown="False" "Brushed Speed" {
          tunnel: w594 -> [w615 w617]
          tunnel: [w612 w616] -> w595
          tunnel: w590 -> [w611 _]
          tunnel: "Min Window" -> [w614 _]
          tunnel: "Max Window" -> [w613 _]
          frame True {
            n270 = To Double Precision Float(number=w611) -> (double precision float=w610:dbl)
            n271 = call "GetSpeed.vi"("Max Window"=w613, "Min Window"=w614, "Y"=w615, "comm seg"=w610) -> ("Speed"=w612:dbl)  [unwired: 6 in, 1 out]
          }
          frame False {
            n272 = call "Brushless Speed Calc (RT).vi"("Data In"=w617) -> ("Speed"=w616:dbl)  [unwired: 14 in]
          }
        }
        "Speed" <- w595
      }
    }
    frame Disabled {
      n273 = while {
        tunnel: w619 -> [w646]
        shift-right: [w639] -> _
        shift-left: _ -> [w638]
        shift-right: [w620] -> _
        shift-left: w618 -> [w622]
        stop <- FALSE stop-if-true
        w634 = 100 ("sample length")
        n274 = local read "Set Threshold"() -> (w644:bool)
        n275 = local read "CommSegs"() -> (w643:i32)
        n276 = local read "Hysteresis"() -> (w645:fxp<+,10,6>)
        n277 = local read "Threshold"() -> (w642:fxp<+/-,24,7>)
        n278 = local read "CtCuttoff"() -> (w641:fxp<+,24,5>)
        n279 = xnode "Read/Write Control"("FPGA VI Reference In"=w646, "Hysteresis"=w645, "Set Threshold"=w644, "CommSegs"=w643, "Threshold level"=w642, "CtCuttoff"=w641) -> ("DataCluster"=w631:T18)  [unwired: 1 in, 2 out]
        n280 = Wait (ms)(milliseconds to wait=u32 10) -> ()  [unwired: 1 out]
        n281 = Tick Count (ms)() -> (millisecond timer value=w639:u32)
        n282 = Cluster To Array(cluster=w631) -> (array=w640:fxp<+/-,25,15>[])
        n283 = Unbundle By Name(w631) -> ("Controller Voltage"=w632:fxp<+/-,25,15>, "Pressure"=w633:fxp<+/-,25,15>)
        n284 = Subtract(x=w639, y=w638) -> (x-y=→"x-y":u32)
        n285 = To Double Precision Float(number=w640) -> (double precision float=w630:dbl[])
        n286 = To Double Precision Float(number=w632) -> (double precision float=w621:dbl)
        n287 = while {
          tunnel: w622 -> [w652]
          tunnel: w621 -> [w648]
          tunnel: [w647] -> w620
          stop <- TRUE stop-if-true
          n288 = Rotate 1D Array(1:w652, 2:1 ("n")) -> (0:w650:dbl[])
          n289 = Insert Into Array(array=w650, index=0, new element=w648) -> (w647:dbl[])
          n290 = call-poly <vilib>:"Butterworth Filter.vi"("high cutoff freq: fh"=10.0, "sampling freq: fs"=100.0, "X"=w647) -> ("Filtered X"=w655:dbl[])  [unwired: 5 in, 1 out]
          n291 = Index Array(array=w655, index=4) -> (element=→"element":dbl)
        }
        n292 = To Double Precision Float(number=w633) -> (double precision float=w635:dbl)
        n293 = call <vilib>:"Mean PtByPt.vi"("x"=w621, "sample length"=w634) -> ("mean"=w628:dbl)  [unwired: 2 in, 1 out]
        n294 = call <vilib>:"Mean PtByPt.vi"("x"=w635, "sample length"=w634) -> ("mean"=w627:dbl)  [unwired: 2 in, 1 out]
        n295 = Replace Array Subset(array=w630, new element=w628, index=5) -> (w629:dbl[])
        n296 = Replace Array Subset(array=w629, new element=w627, index=2) -> (→"output array":dbl[])
      }
    }
  }
  n297 = call "CAN Communication.vi"("CAN Mode"=CAN_Mode."Init", "Error IN"=w25) -> ("Error OUT"=w19:errorcluster)  [unwired: 8 in, 1 out]
  n298 = call "RT Engine.vi"("Error In"=w25) -> ()  [unwired: 11 in]
  n299 = flat-sequence {
    tunnel: w15 -> [w659]
    frame #0 {
      n300 = Wait on Occurrence(2:w659) -> ()  [unwired: 2 in, 1 out]
    }
    frame #1 {
      n301 = call "AI RT FIFO.vi"("Mode"=Stream_RT_FIFO_Mode."Create", "Buffer Size"=800, "# of elements"=8) -> ()  [unwired: 10 in, 3 out]
    }
    frame #2 {
      n302 = control-ref of="Stream Stop"() -> (w665:refnum<vi>)
      n303 = property class="Bool (strict)"(reference=w665, "Value"=FALSE) -> (reference out=w663:refnum<vi>)  [unwired: 1 in, 1 out]
      n304 = call "Loop (Data Stream).vi"("Stop"=w663) -> ()  [unwired: 10 in, 1 out]
    }
    frame #3 {
      n305 = call "AI RT FIFO.vi"("Mode"=Stream_RT_FIFO_Mode."Delete") -> ()  [unwired: 12 in, 3 out]
    }
  }
  n306 = while {
    tunnel: w19 -> [w673]
    i -> [w672]
    stop <- FALSE stop-if-true
    n307 = local read "Controller Name"() -> (w674:T5)
    n308 = Quotient & Remainder(x=w672, y=10) -> (x-y*floor(x/y)=w670:i32)  [unwired: 1 out]
    n309 = Equal To 0?(x=w670) -> (x = 0?=w669:bool)
    n310 = case shown="\"Conti\"" w674 {
      tunnel: w673 -> [_ w677 w680 w683 w686 w688 w690]
      tunnel: w669 -> [_ _ w679 _ _ _ _]
      tunnel: "CAN CMD" -> [_ w676 w678 w681 w685 w687 w689]
      frame Default {
        n311 = Wait (ms)(milliseconds to wait=u32 500) -> ()  [unwired: 1 out]
      }
      frame "Conti" {
        n312 = call "Conti CAN.vi"("Error IN"=w677, "CMD"=w676) -> ()  [unwired: 9 in, 1 out]
      }
      frame "Helbako (old)" {
        n313 = call "Helbako CAN.vi"("Split-timer"=w679, "Error IN"=w680, "CMD"=w678) -> ()  [unwired: 8 in, 1 out]
      }
      frame "Hella BLDC Screw" {
        n314 = To Unsigned Byte Integer(number=w681) -> (unsigned 8bit integer=w682:u8)
        n315 = call "Hella CAN.vi"("Error IN"=w683, "CMD"=w682) -> ()  [unwired: 9 in, 1 out]
      }
      frame "Hella BLDC Turbine" {
        n316 = To Unsigned Byte Integer(number=w685) -> (unsigned 8bit integer=w684:u8)
        n317 = call "Hella CAN Turbine.vi"("Error IN"=w686, "CMD"=w684) -> ()  [unwired: 9 in, 1 out]
      }
      frame "Hella Gas" {
        n318 = call "Hella CAN Gas.vi"("Pressure Command (kPa)"=w687, "Error In"=w688) -> ()  [unwired: 12 in, 2 out]
      }
      frame "Hella Diesel" {
        n319 = call "Hella CAN Diesel.vi"("Command (kPa)"=w689, "Error In"=w690) -> ()  [unwired: 13 in, 1 out]
      }
    }
  }
